vi "VI Server_Set Controls Property from String Formats.vi"(6 "Defer Panel Updates (T)":bool=TRUE, 7 "Property (Value)":T2="Value", 8 "error in (no error)":errorcluster, 9 "New Values":string[](array[string]), 10 "Labels":string[](array[string]), 11 "VI Server Cluster":T1={"Labels"=["Label", "Size", "Font", "Heght", "Width", "Ledding Denominator", "Ledding Nominator", "Label Number", "Microstep Resolution", "X", "Y", "Z", "Italic?", "Underlined?"], "Refs"=[], "VI Ref"=refnum}) -> (0 "error out":errorcluster, 2 "Labels.Text":string[](array[string]), 3 "VI Server Cluster.DUP":T1={"Labels"=["Label", "Size", "Font", "Heght", "Width", "Ledding Denominator", "Ledding Nominator", "Label Number", "Microstep Resolution", "X", "Y", "Z", "Italic?", "Underlined?"], "Refs"=[], "VI Ref"=refnum})   [LabVIEW 2020, in "VI Server Toolkit LV2013.lvlib"]
doc: "Set multiple controls <B>Property</B> from string equivalents.\nList of properties include (if applicable):\n- Value;\n- Format;\n-Format String;\n- Increment;\n-Minimum;\n-Maximum;\n-Precision;\n-Boolean Text;\n-Caption."
uses:
  VI Server Toolkit LV2013.lvlib
  VI Server_TypeDefs/VI Server_RefsCluster.ctl
  VI Server Libraries/VI Server Controls.llb/VI Server_Properties.ctl
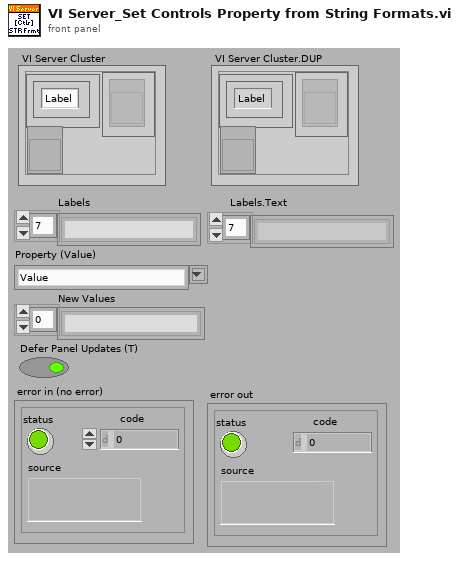
[diagram p1: front panel]
types:
  T1 = typedef "VI Server_RefsCluster.ctl" = cluster{"Labels":string[], "Refs":refnum<vi>[], "VI Ref":refnum<vi>}
  T2 = typedef "VI Server Toolkit LV2013.lvlib/VI Server_Properties.ctl" = string
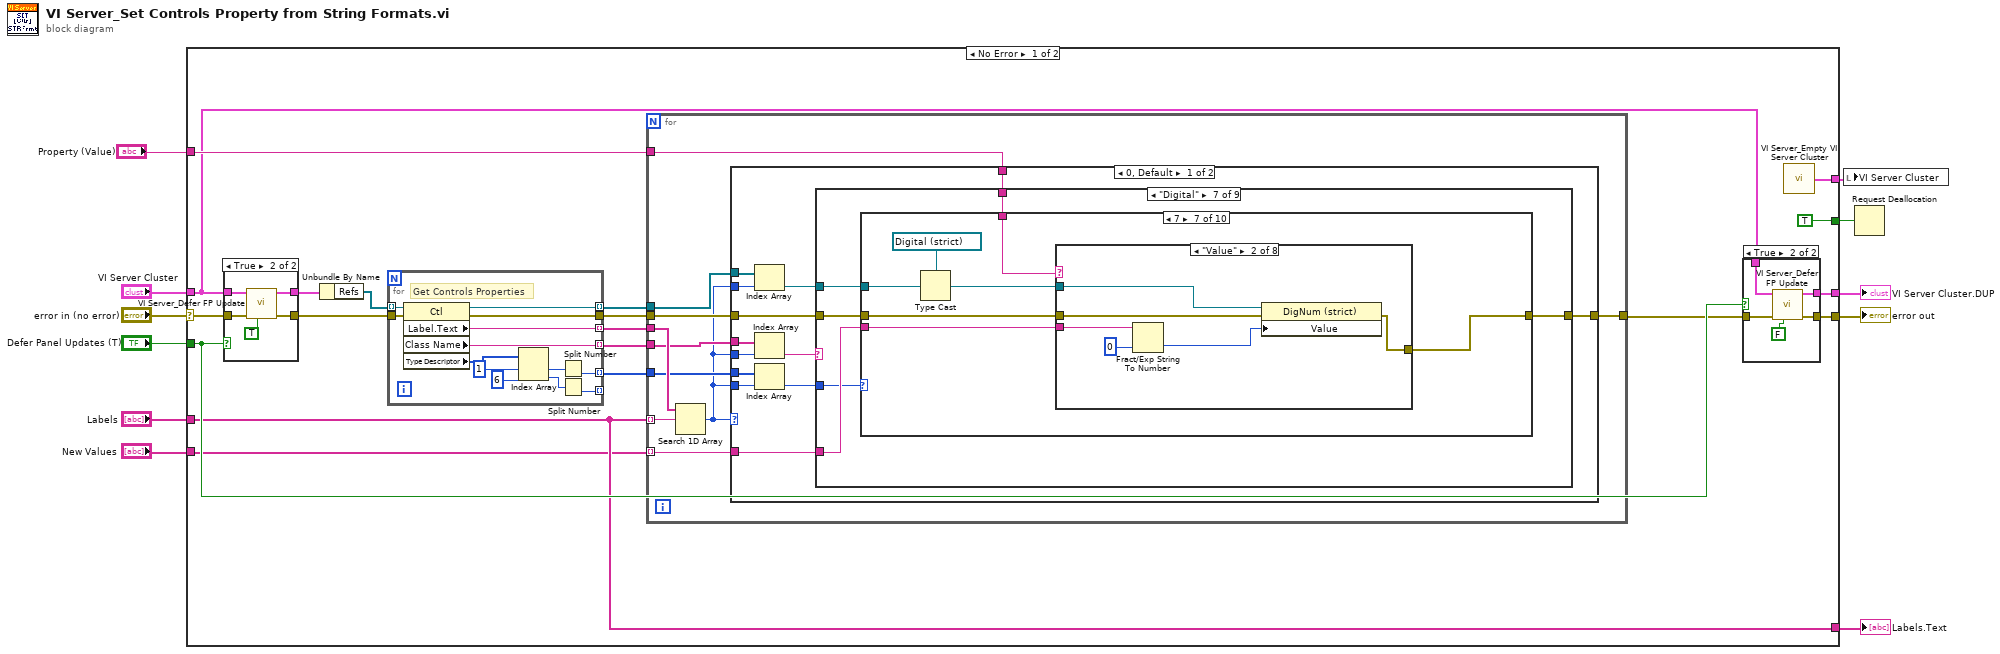
[diagram p0: block diagram]
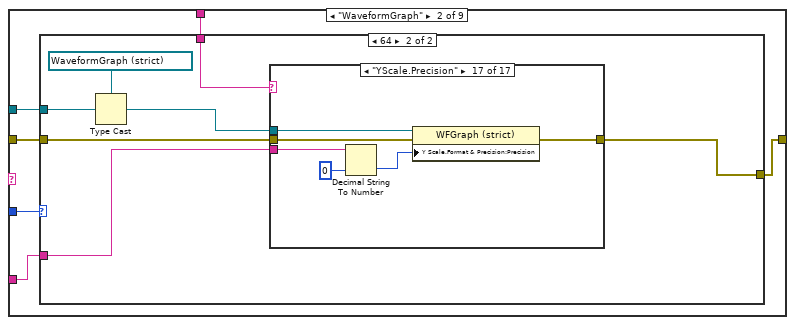
[diagram p3: hidden frame]
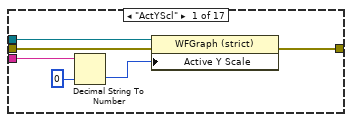
[diagram p5: hidden frame]
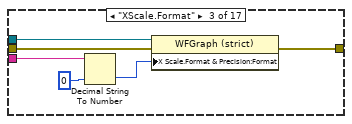
[diagram p7: hidden frame]
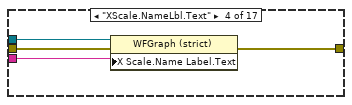
[diagram p8: hidden frame]
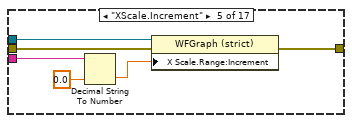
[diagram p9: hidden frame]
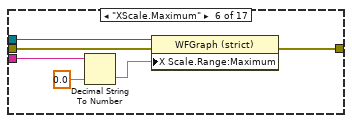
[diagram p10: hidden frame]
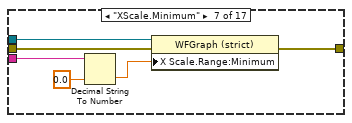
[diagram p11: hidden frame]
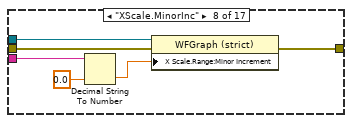
[diagram p12: hidden frame]
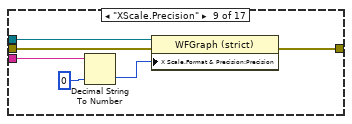
[diagram p13: hidden frame]
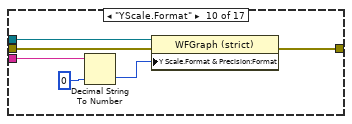
[diagram p14: hidden frame]
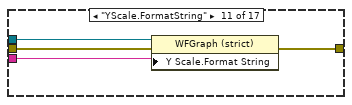
[diagram p15: hidden frame]
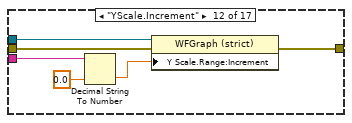
[diagram p16: hidden frame]
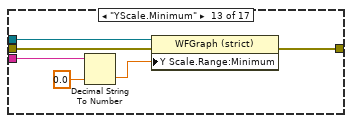
[diagram p17: hidden frame]
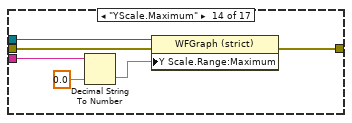
[diagram p18: hidden frame]
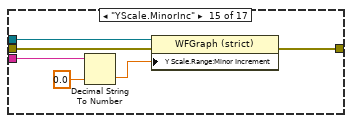
[diagram p19: hidden frame]
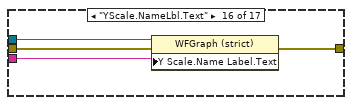
[diagram p20: hidden frame]
diagram:
  n1 = case shown="No Error" "error in (no error)" {
    selector: "error in (no error)" -> [w29 w1413]
    tunnel: "Labels" -> [w15 _]
    tunnel: "New Values" -> [w14 _]
    tunnel: [w26 w1413] -> w9
    tunnel: "VI Server Cluster" -> [w13 _]
    tunnel: "Property (Value)" -> [w19 _]
    tunnel: [w15 _] -> w5
    tunnel: [w25 _] -> w4
    tunnel: "Defer Panel Updates (T)" -> [w24 _]
    tunnel: [TRUE _] -> w2
    tunnel: [w12 _] -> w1
    frame No Error {
      n2 = case shown="True" w24 {
        tunnel: w29 -> [w1394 w1399]
        tunnel: [w1394 w1398] -> w28
        tunnel: w13 -> [w1393 w1397]
        tunnel: [w1393 w1396] -> w27
        frame False {
        }
        frame True {
          n3 = call "VI Server_Defer FP Update.vi"("Defer Panel Updates? (F)"=TRUE ("Defer Panel Updates (F)"), "error in"=w1399, "VI Server Cluster"=w1397) -> ("error out"=w1398:errorcluster, "VI Server Cluster.DUP"=w1396:T1)  [unwired: 7 out]
        }
      }
      n4 = Unbundle By Name(w27) -> ("Refs"=w30:refnum<vi>[])
      n5 = for {
        tunnel: w30 -> [w1412] mode=indexing
        tunnel: w28 -> [w1411]
        tunnel: [w1410] -> w20 mode=indexing
        tunnel: [w1409] -> w17 mode=indexing
        tunnel: [w1408] -> w21 mode=indexing
        tunnel: [w1407] -> w22
        tunnel: [w1403] -> w16 mode=indexing
        tunnel: [w1400] -> _ mode=indexing
        # "Get Controls Properties"
        n6 = property class="Ctl"(reference=w1412, error in=w1411) -> (reference out=w1408:refnum<vi>, error out=w1407:errorcluster, "Label.Text"=w1410:string, "Class Name"=w1409:string, "Type Descriptor"=w1406:i16[])
        n7 = Index Array(array=w1406, index #1=1 ("index"), index #2=6 ("index")) -> (element #1=w1404:i16, element #2=w1401:i16)
        n8 = Split Number(x=w1404) -> (lo(x)=w1403:u8)  [unwired: 1 out]
        n9 = Split Number(x=w1401) -> (lo(x)=w1400:u8)  [unwired: 1 out]
      }
      n10 = for {
        tunnel: w15 -> [w38] mode=indexing
        tunnel: w20 -> [w40]
        tunnel: w21 -> [w36]
        tunnel: w17 -> [w39]
        tunnel: w14 -> [w37] mode=indexing
        tunnel: w22 -> [w35]
        tunnel: [w34] -> w18
        tunnel: w16 -> [w33]
        tunnel: w19 -> [w31]
        n11 = Search 1D Array(1D array=w40, element=w38) -> (index of element=w32:i32)  [unwired: 1 out]
        n12 = case shown="0, Default" w32 {
          tunnel: w36 -> [w53 _]
          tunnel: w32 -> [w52 _]
          tunnel: w39 -> [w51 _]
          tunnel: w32 -> [w50 _]
          tunnel: w37 -> [w47 _]
          tunnel: w35 -> [w46 w1385]
          tunnel: [w45 w1385] -> w34
          tunnel: w33 -> [w44 _]
          tunnel: w32 -> [w43 _]
          tunnel: w31 -> [w41 _]
          frame 0, Default {
            n13 = Index Array(array=w53, index=w52) -> (element=w48:refnum<vi>)
            n14 = Index Array(array=w51, index=w50) -> (element=w49:string)
            n15 = Index Array(array=w44, index=w43) -> (element=w42:u8)
            n16 = case shown="\"Digital\"" w49 {
              tunnel: w48 -> [_ w58 w162 w170 w182 w191 w195 w661 w1371]
              tunnel: w47 -> [_ w56 w167 w178 w185 w189 w194 w660 w1369]
              tunnel: w46 -> [w54 w59 w165 w173 w183 w188 w197 w663 w1373]
              tunnel: [w54 w55 w163 w171 w184 w187 w196 w662 w1372] -> w45
              tunnel: w42 -> [_ w60 _ _ _ _ w193 w659 _]
              tunnel: w41 -> [_ w57 _ _ _ _ w192 w658 w1367]
              frame "", Default {
              }
              frame "WaveformGraph" {
                n17 = case shown="64" w60 {
                  tunnel: w59 -> [w61 w65]
                  tunnel: w58 -> [_ w68]
                  tunnel: w57 -> [_ w64]
                  tunnel: w56 -> [_ w63]
                  tunnel: [w61 w62] -> w55
                  frame 0, Default {
                  }
                  frame 64 {
                    n18 = Type Cast(type=refnum<vi> refnum ("XY Graph"), x=w68) -> (*(type *) &x=w66:refnum<vi>)
                    n19 = case shown="\"YScale.Precision\"" w64 {
                      tunnel: w66 -> [w74 _ w81 w85 w91 w97 w103 w109 w115 w121 w125 w131 w137 w143 w149 w153 w159]
                      tunnel: w65 -> [w73 w75 w80 w84 w90 w96 w102 w108 w114 w120 w124 w130 w136 w142 w148 w152 w158]
                      tunnel: w63 -> [w72 _ w78 w82 w88 w94 w100 w106 w112 w118 w122 w128 w134 w140 w146 w150 w156]
                      tunnel: [w71 w75 w79 w83 w89 w95 w101 w107 w113 w119 w123 w129 w135 w141 w147 w151 w157] -> w62
                      frame "ActYScl" {
                        n20 = Decimal String To Number(string=w72, default (0L)=0 ("Active Y Scale")) -> (number=w69:i32)  [unwired: 2 out]
                        n21 = property class="WFGraph (strict)"(reference=w74, error in=w73, "Active Y Scale"=w69) -> (error out=w71:errorcluster)  [unwired: 1 out]
                      }
                      frame "False", Default {
                      }
                      frame "XScale.Format" {
                        n22 = Decimal String To Number(string=w78, default (0L)=u8 0 ("Y Scale.Format & Precision:Format")) -> (number=w77:u8)  [unwired: 2 out]
                        n23 = property class="WFGraph (strict)"(reference=w81, error in=w80, "X Scale.Format & Precision:Format"=w77) -> (error out=w79:errorcluster)  [unwired: 1 out]
                      }
                      frame "XScale.NameLbl.Text" {
                        n24 = property class="WFGraph (strict)"(reference=w85, error in=w84, "X Scale.Name Label.Text"=w82) -> (error out=w83:errorcluster)  [unwired: 1 out]
                      }
                      frame "XScale.Increment" {
                        n25 = Decimal String To Number(string=w88, default (0L)=0.0 ("X Scale.Range:Minimum")) -> (number=w86:dbl)  [unwired: 2 out]
                        n26 = property class="WFGraph (strict)"(reference=w91, error in=w90, "X Scale.Range:Increment"=w86) -> (error out=w89:errorcluster)  [unwired: 1 out]
                      }
                      frame "XScale.Maximum" {
                        n27 = Decimal String To Number(string=w94, default (0L)=0.0 ("X Scale.Range:Minimum")) -> (number=w92:dbl)  [unwired: 2 out]
                        n28 = property class="WFGraph (strict)"(reference=w97, error in=w96, "X Scale.Range:Maximum"=w92) -> (error out=w95:errorcluster)  [unwired: 1 out]
                      }
                      frame "XScale.Minimum" {
                        n29 = Decimal String To Number(string=w100, default (0L)=0.0 ("X Scale.Range:Minimum")) -> (number=w98:dbl)  [unwired: 2 out]
                        n30 = property class="WFGraph (strict)"(reference=w103, error in=w102, "X Scale.Range:Minimum"=w98) -> (error out=w101:errorcluster)  [unwired: 1 out]
                      }
                      frame "XScale.MinorInc" {
                        n31 = Decimal String To Number(string=w106, default (0L)=0.0 ("X Scale.Range:Minimum")) -> (number=w104:dbl)  [unwired: 2 out]
                        n32 = property class="WFGraph (strict)"(reference=w109, error in=w108, "X Scale.Range:Minor Increment"=w104) -> (error out=w107:errorcluster)  [unwired: 1 out]
                      }
                      frame "XScale.Precision" {
                        n33 = Decimal String To Number(string=w112, default (0L)=u8 0 ("Y Scale.Format & Precision:Format")) -> (number=w111:u8)  [unwired: 2 out]
                        n34 = property class="WFGraph (strict)"(reference=w115, error in=w114, "X Scale.Format & Precision:Precision"=w111) -> (error out=w113:errorcluster)  [unwired: 1 out]
                      }
                      frame "YScale.Format" {
                        n35 = Decimal String To Number(string=w118, default (0L)=u8 0 ("Y Scale.Format & Precision:Format")) -> (number=w117:u8)  [unwired: 2 out]
                        n36 = property class="WFGraph (strict)"(reference=w121, error in=w120, "Y Scale.Format & Precision:Format"=w117) -> (error out=w119:errorcluster)  [unwired: 1 out]
                      }
                      frame "YScale.FormatString" {
                        n37 = property class="WFGraph (strict)"(reference=w125, error in=w124, "Y Scale.Format String"=w122) -> (error out=w123:errorcluster)  [unwired: 1 out]
                      }
                      frame "YScale.Increment" {
                        n38 = Decimal String To Number(string=w128, default (0L)=0.0 ("X Scale.Range:Minimum")) -> (number=w126:dbl)  [unwired: 2 out]
                        n39 = property class="WFGraph (strict)"(reference=w131, error in=w130, "Y Scale.Range:Increment"=w126) -> (error out=w129:errorcluster)  [unwired: 1 out]
                      }
                      frame "YScale.Minimum" {
                        n40 = Decimal String To Number(string=w134, default (0L)=0.0 ("X Scale.Range:Minimum")) -> (number=w132:dbl)  [unwired: 2 out]
                        n41 = property class="WFGraph (strict)"(reference=w137, error in=w136, "Y Scale.Range:Minimum"=w132) -> (error out=w135:errorcluster)  [unwired: 1 out]
                      }
                      frame "YScale.Maximum" {
                        n42 = Decimal String To Number(string=w140, default (0L)=0.0 ("X Scale.Range:Minimum")) -> (number=w138:dbl)  [unwired: 2 out]
                        n43 = property class="WFGraph (strict)"(reference=w143, error in=w142, "Y Scale.Range:Maximum"=w138) -> (error out=w141:errorcluster)  [unwired: 1 out]
                      }
                      frame "YScale.MinorInc" {
                        n44 = Decimal String To Number(string=w146, default (0L)=0.0 ("X Scale.Range:Minimum")) -> (number=w144:dbl)  [unwired: 2 out]
                        n45 = property class="WFGraph (strict)"(reference=w149, error in=w148, "Y Scale.Range:Minor Increment"=w144) -> (error out=w147:errorcluster)  [unwired: 1 out]
                      }
                      frame "YScale.NameLbl.Text" {
                        n46 = property class="WFGraph (strict)"(reference=w153, error in=w152, "Y Scale.Name Label.Text"=w150) -> (error out=w151:errorcluster)  [unwired: 1 out]
                      }
                      frame "YScale.Precision" {
                        n47 = Decimal String To Number(string=w156, default (0L)=u8 0 ("Y Scale.Format & Precision:Format")) -> (number=w155:u8)  [unwired: 2 out]
                        n48 = property class="WFGraph (strict)"(reference=w159, error in=w158, "Y Scale.Format & Precision:Precision"=w155) -> (error out=w157:errorcluster)  [unwired: 1 out]
                      }
                    }
                  }
                }
              }
              frame "Enum" {
                n49 = Type Cast(type=refnum<vi> refnum ("Enum"), x=w162) -> (*(type *) &x=w168:refnum<vi>)
                n50 = property class="Enum (strict)"(reference=w168, error in=w165) -> (error out=w164:errorcluster, "Strings []"=w166:string[])  [unwired: 1 out]
                n51 = Search 1D Array(1D array=w166, element=w167) -> (index of element=w161:i32)  [unwired: 1 out]
                n52 = To Variant(anything=w161) -> (Variant=w160:variant)
                n53 = property class="Ctl"(reference=w162, error in=w164, "Value"=w160) -> (error out=w163:errorcluster)  [unwired: 1 out]
              }
              frame "Ring" {
                n54 = Type Cast(type=refnum<vi> refnum ("Ring"), x=w170) -> (*(type *) &x=w179:refnum<vi>)
                n55 = property class="Ring (strict)"(reference=w179, error in=w173) -> (error out=w172:errorcluster, "Strings []"=w176:string[])  [unwired: 1 out]
                n56 = Search 1D Array(1D array=w176, element=w178) -> (index of element=w177:i32)  [unwired: 1 out]
                n57 = To Variant(anything=w177) -> (Variant=w175:variant)
                n58 = property class="Ctl"(reference=w170, error in=w172, "Value"=w175) -> (error out=w171:errorcluster)  [unwired: 1 out]
              }
              frame "Path" {
                n59 = String To Path(string=w185) -> (path=w186:path)
                n60 = Type Cast(type=refnum<vi> refnum ("Path"), x=w182) -> (*(type *) &x=w181:refnum<vi>)
                n61 = property class="Path"(reference=w181, error in=w183, "Value"=w186) -> (error out=w184:errorcluster)  [unwired: 1 out]
              }
              frame "String" {
                n62 = To Variant(anything=w189) -> (Variant=w190:variant)
                n63 = property class="Ctl"(reference=w191, error in=w188, "Value"=w190) -> (error out=w187:errorcluster)  [unwired: 1 out]
              }
              frame "Digital" {
                n64 = case shown="7" w193 {
                  tunnel: w197 -> [w198 w205 w254 w298 w350 w397 w450 w498 w548 w608]
                  tunnel: [w198 w204 w250 w300 w353 w399 w448 w496 w550 w607] -> w196
                  tunnel: w195 -> [_ w203 w256 w304 w355 w403 w454 w502 w554 w612]
                  tunnel: w194 -> [_ w201 w253 w299 w349 w398 w449 w497 w549 w606]
                  tunnel: w192 -> [_ w199 w252 w302 w352 w401 w452 w499 w552 w610]
                  frame 0, Default {
                  }
                  frame 1 {
                    n65 = Type Cast(type=refnum<vi> refnum ("I8"), x=w203) -> (*(type *) &x=w202:refnum<vi>)
                    n66 = case shown="\"Value\"" w199 {
                      tunnel: w205 -> [w206 w212 w218 w225 w232 w237 w243 w249]
                      tunnel: [w206 w211 w217 w224 w231 w236 w242 w248] -> w204
                      tunnel: w202 -> [_ w210 w216 w223 w230 w235 w241 w247]
                      tunnel: w201 -> [_ w208 w215 w222 w229 w234 w240 w246]
                      frame "False", Default {
                      }
                      frame "Value" {
                        n67 = Fract/Exp String To Number(string=w208, default (0 dbl)=i8 0) -> (number=w207:i8)  [unwired: 3 out]
                        n68 = property class="DigNum (strict)"(reference=w210, error in=w212, "Value"=w207) -> (error out=w211:errorcluster)  [unwired: 1 out]
                      }
                      frame "Minimum" {
                        n69 = Fract/Exp String To Number(string=w215, default (0 dbl)=0.0 ("Data Range:Minimum")) -> (number=w213:dbl)  [unwired: 3 out]
                        n70 = property class="DigNum (strict)"(reference=w216, error in=w218, "Data Range:Minimum"=w213) -> (reference out=w219:refnum<vi>, error out=w217:errorcluster)
                        n71 = Close Reference(reference=w219) -> ()  [unwired: 1 in, 1 out]
                      }
                      frame "Maximum" {
                        n72 = Fract/Exp String To Number(string=w222, default (0 dbl)=0.0 ("Data Range:Minimum")) -> (number=w220:dbl)  [unwired: 3 out]
                        n73 = property class="DigNum (strict)"(reference=w223, error in=w225, "Data Range:Maximum"=w220) -> (reference out=w226:refnum<vi>, error out=w224:errorcluster)
                        n74 = Close Reference(reference=w226) -> ()  [unwired: 1 in, 1 out]
                      }
                      frame "Increment" {
                        n75 = Fract/Exp String To Number(string=w229, default (0 dbl)=0.0 ("Data Range:Minimum")) -> (number=w227:dbl)  [unwired: 3 out]
                        n76 = property class="DigNum (strict)"(reference=w230, error in=w232, "Data Range:Increment"=w227) -> (reference out=w233:refnum<vi>, error out=w231:errorcluster)
                        n77 = Close Reference(reference=w233) -> ()  [unwired: 1 in, 1 out]
                      }
                      frame "Format String" {
                        n78 = property class="DigNum (strict)"(reference=w235, error in=w237, "Format String"=w234) -> (error out=w236:errorcluster)  [unwired: 1 out]
                      }
                      frame "Format" {
                        n79 = Decimal String To Number(string=w240, default (0L)=u8 0 ("Format & Precision:Format")) -> (number=w238:u8)  [unwired: 2 out]
                        n80 = property class="DigNum (strict)"(reference=w241, error in=w243, "Format & Precision:Format"=w238) -> (error out=w242:errorcluster)  [unwired: 1 out]
                      }
                      frame "Precision" {
                        n81 = Decimal String To Number(string=w246, default (0L)=u8 0 ("Format & Precision:Format")) -> (number=w244:u8)  [unwired: 2 out]
                        n82 = property class="DigNum (strict)"(reference=w247, error in=w249, "Format & Precision:Precision"=w244) -> (error out=w248:errorcluster)  [unwired: 1 out]
                      }
                    }
                  }
                  frame 2 {
                    n83 = Type Cast(type=refnum<vi> refnum ("I16"), x=w256) -> (*(type *) &x=w251:refnum<vi>)
                    n84 = case shown="\"Value\"" w252 {
                      tunnel: w254 -> [w257 w263 w269 w275 w281 w285 w291 w297]
                      tunnel: [w257 w262 w268 w274 w280 w284 w290 w296] -> w250
                      tunnel: w251 -> [_ w261 w267 w273 w279 w283 w289 w295]
                      tunnel: w253 -> [_ w260 w266 w272 w278 w282 w288 w294]
                      frame "False", Default {
                      }
                      frame "Value" {
                        n85 = Fract/Exp String To Number(string=w260, default (0 dbl)=i16 0) -> (number=w259:i16)  [unwired: 3 out]
                        n86 = property class="DigNum (strict)"(reference=w261, error in=w263, "Value"=w259) -> (error out=w262:errorcluster)  [unwired: 1 out]
                      }
                      frame "Minimum" {
                        n87 = Fract/Exp String To Number(string=w266, default (0 dbl)=0.0 ("Data Range:Minimum")) -> (number=w264:dbl)  [unwired: 3 out]
                        n88 = property class="DigNum (strict)"(reference=w267, error in=w269, "Data Range:Minimum"=w264) -> (error out=w268:errorcluster)  [unwired: 1 out]
                      }
                      frame "Maximum" {
                        n89 = Fract/Exp String To Number(string=w272, default (0 dbl)=0.0 ("Data Range:Minimum")) -> (number=w270:dbl)  [unwired: 3 out]
                        n90 = property class="DigNum (strict)"(reference=w273, error in=w275, "Data Range:Maximum"=w270) -> (error out=w274:errorcluster)  [unwired: 1 out]
                      }
                      frame "Increment" {
                        n91 = Fract/Exp String To Number(string=w278, default (0 dbl)=0.0 ("Data Range:Minimum")) -> (number=w276:dbl)  [unwired: 3 out]
                        n92 = property class="DigNum (strict)"(reference=w279, error in=w281, "Data Range:Increment"=w276) -> (error out=w280:errorcluster)  [unwired: 1 out]
                      }
                      frame "Format String" {
                        n93 = property class="DigNum (strict)"(reference=w283, error in=w285, "Format String"=w282) -> (error out=w284:errorcluster)  [unwired: 1 out]
                      }
                      frame "Format" {
                        n94 = Decimal String To Number(string=w288, default (0L)=u8 0 ("Format & Precision:Format")) -> (number=w286:u8)  [unwired: 2 out]
                        n95 = property class="DigNum (strict)"(reference=w289, error in=w291, "Format & Precision:Format"=w286) -> (error out=w290:errorcluster)  [unwired: 1 out]
                      }
                      frame "Precision" {
                        n96 = Decimal String To Number(string=w294, default (0L)=u8 0 ("Format & Precision:Format")) -> (number=w292:u8)  [unwired: 2 out]
                        n97 = property class="DigNum (strict)"(reference=w295, error in=w297, "Format & Precision:Precision"=w292) -> (error out=w296:errorcluster)  [unwired: 1 out]
                      }
                    }
                  }
                  frame 3 {
                    n98 = Type Cast(type=refnum<vi> refnum ("I32"), x=w304) -> (*(type *) &x=w301:refnum<vi>)
                    n99 = case shown="\"Value\"" w302 {
                      tunnel: w298 -> [w305 w311 w317 w324 w331 w336 w342 w348]
                      tunnel: [w305 w310 w316 w323 w330 w335 w341 w347] -> w300
                      tunnel: w301 -> [_ w309 w315 w322 w329 w334 w340 w346]
                      tunnel: w299 -> [_ w308 w314 w321 w328 w333 w339 w345]
                      frame "False", Default {
                      }
                      frame "Value" {
                        n100 = Fract/Exp String To Number(string=w308, default (0 dbl)=0) -> (number=w307:i32)  [unwired: 3 out]
                        n101 = property class="DigNum (strict)"(reference=w309, error in=w311, "Value"=w307) -> (error out=w310:errorcluster)  [unwired: 1 out]
                      }
                      frame "Minimum" {
                        n102 = Fract/Exp String To Number(string=w314, default (0 dbl)=0.0 ("Data Range:Minimum")) -> (number=w312:dbl)  [unwired: 3 out]
                        n103 = property class="DigNum (strict)"(reference=w315, error in=w317, "Data Range:Minimum"=w312) -> (reference out=w318:refnum<vi>, error out=w316:errorcluster)
                        n104 = Close Reference(reference=w318) -> ()  [unwired: 1 in, 1 out]
                      }
                      frame "Maximum" {
                        n105 = Fract/Exp String To Number(string=w321, default (0 dbl)=0.0 ("Data Range:Minimum")) -> (number=w319:dbl)  [unwired: 3 out]
                        n106 = property class="DigNum (strict)"(reference=w322, error in=w324, "Data Range:Maximum"=w319) -> (reference out=w325:refnum<vi>, error out=w323:errorcluster)
                        n107 = Close Reference(reference=w325) -> ()  [unwired: 1 in, 1 out]
                      }
                      frame "Increment" {
                        n108 = Fract/Exp String To Number(string=w328, default (0 dbl)=0.0 ("Data Range:Minimum")) -> (number=w326:dbl)  [unwired: 3 out]
                        n109 = property class="DigNum (strict)"(reference=w329, error in=w331, "Data Range:Increment"=w326) -> (reference out=w332:refnum<vi>, error out=w330:errorcluster)
                        n110 = Close Reference(reference=w332) -> ()  [unwired: 1 in, 1 out]
                      }
                      frame "Format String" {
                        n111 = property class="DigNum (strict)"(reference=w334, error in=w336, "Format String"=w333) -> (error out=w335:errorcluster)  [unwired: 1 out]
                      }
                      frame "Format" {
                        n112 = Decimal String To Number(string=w339, default (0L)=u8 0 ("Format & Precision:Format")) -> (number=w337:u8)  [unwired: 2 out]
                        n113 = property class="DigNum (strict)"(reference=w340, error in=w342, "Format & Precision:Format"=w337) -> (error out=w341:errorcluster)  [unwired: 1 out]
                      }
                      frame "Precision" {
                        n114 = Decimal String To Number(string=w345, default (0L)=u8 0 ("Format & Precision:Format")) -> (number=w343:u8)  [unwired: 2 out]
                        n115 = property class="DigNum (strict)"(reference=w346, error in=w348, "Format & Precision:Precision"=w343) -> (error out=w347:errorcluster)  [unwired: 1 out]
                      }
                    }
                  }
                  frame 5 {
                    n116 = Type Cast(type=refnum<vi> refnum ("U8"), x=w355) -> (*(type *) &x=w351:refnum<vi>)
                    n117 = case shown="\"Value\"" w352 {
                      tunnel: w350 -> [w356 w362 w368 w374 w380 w384 w390 w396]
                      tunnel: [w356 w361 w367 w373 w379 w383 w389 w395] -> w353
                      tunnel: w351 -> [_ w360 w366 w372 w378 w382 w388 w394]
                      tunnel: w349 -> [_ w359 w365 w371 w377 w381 w387 w393]
                      frame "False", Default {
                      }
                      frame "Value" {
                        n118 = Fract/Exp String To Number(string=w359, default (0 dbl)=u8 0) -> (number=w358:u8)  [unwired: 3 out]
                        n119 = property class="DigNum (strict)"(reference=w360, error in=w362, "Value"=w358) -> (error out=w361:errorcluster)  [unwired: 1 out]
                      }
                      frame "Minimum" {
                        n120 = Fract/Exp String To Number(string=w365, default (0 dbl)=0.0 ("Data Range:Minimum")) -> (number=w363:dbl)  [unwired: 3 out]
                        n121 = property class="DigNum (strict)"(reference=w366, error in=w368, "Data Range:Minimum"=w363) -> (error out=w367:errorcluster)  [unwired: 1 out]
                      }
                      frame "Maximum" {
                        n122 = Fract/Exp String To Number(string=w371, default (0 dbl)=0.0 ("Data Range:Minimum")) -> (number=w369:dbl)  [unwired: 3 out]
                        n123 = property class="DigNum (strict)"(reference=w372, error in=w374, "Data Range:Maximum"=w369) -> (error out=w373:errorcluster)  [unwired: 1 out]
                      }
                      frame "Increment" {
                        n124 = Fract/Exp String To Number(string=w377, default (0 dbl)=0.0 ("Data Range:Minimum")) -> (number=w375:dbl)  [unwired: 3 out]
                        n125 = property class="DigNum (strict)"(reference=w378, error in=w380, "Data Range:Increment"=w375) -> (error out=w379:errorcluster)  [unwired: 1 out]
                      }
                      frame "Format String" {
                        n126 = property class="DigNum (strict)"(reference=w382, error in=w384, "Format String"=w381) -> (error out=w383:errorcluster)  [unwired: 1 out]
                      }
                      frame "Format" {
                        n127 = Decimal String To Number(string=w387, default (0L)=u8 0 ("Format & Precision:Format")) -> (number=w385:u8)  [unwired: 2 out]
                        n128 = property class="DigNum (strict)"(reference=w388, error in=w390, "Format & Precision:Format"=w385) -> (error out=w389:errorcluster)  [unwired: 1 out]
                      }
                      frame "Precision" {
                        n129 = Decimal String To Number(string=w393, default (0L)=u8 0 ("Format & Precision:Format")) -> (number=w391:u8)  [unwired: 2 out]
                        n130 = property class="DigNum (strict)"(reference=w394, error in=w396, "Format & Precision:Precision"=w391) -> (error out=w395:errorcluster)  [unwired: 1 out]
                      }
                    }
                  }
                  frame 6 {
                    n131 = Type Cast(type=refnum<vi> refnum ("U16"), x=w403) -> (*(type *) &x=w400:refnum<vi>)
                    n132 = case shown="\"Value\"" w401 {
                      tunnel: w397 -> [w404 w410 w416 w423 w430 w435 w441 w447]
                      tunnel: [w404 w409 w415 w422 w429 w434 w440 w446] -> w399
                      tunnel: w400 -> [_ w408 w414 w421 w428 w433 w439 w445]
                      tunnel: w398 -> [_ w407 w413 w420 w427 w432 w438 w444]
                      frame "False", Default {
                      }
                      frame "Value" {
                        n133 = Fract/Exp String To Number(string=w407, default (0 dbl)=u16 0) -> (number=w406:u16)  [unwired: 3 out]
                        n134 = property class="DigNum (strict)"(reference=w408, error in=w410, "Value"=w406) -> (error out=w409:errorcluster)  [unwired: 1 out]
                      }
                      frame "Minimum" {
                        n135 = Fract/Exp String To Number(string=w413, default (0 dbl)=0.0 ("Data Range:Minimum")) -> (number=w411:dbl)  [unwired: 3 out]
                        n136 = property class="DigNum (strict)"(reference=w414, error in=w416, "Data Range:Minimum"=w411) -> (reference out=w417:refnum<vi>, error out=w415:errorcluster)
                        n137 = Close Reference(reference=w417) -> ()  [unwired: 1 in, 1 out]
                      }
                      frame "Maximum" {
                        n138 = Fract/Exp String To Number(string=w420, default (0 dbl)=0.0 ("Data Range:Minimum")) -> (number=w418:dbl)  [unwired: 3 out]
                        n139 = property class="DigNum (strict)"(reference=w421, error in=w423, "Data Range:Maximum"=w418) -> (reference out=w424:refnum<vi>, error out=w422:errorcluster)
                        n140 = Close Reference(reference=w424) -> ()  [unwired: 1 in, 1 out]
                      }
                      frame "Increment" {
                        n141 = Fract/Exp String To Number(string=w427, default (0 dbl)=0.0 ("Data Range:Minimum")) -> (number=w425:dbl)  [unwired: 3 out]
                        n142 = property class="DigNum (strict)"(reference=w428, error in=w430, "Data Range:Increment"=w425) -> (reference out=w431:refnum<vi>, error out=w429:errorcluster)
                        n143 = Close Reference(reference=w431) -> ()  [unwired: 1 in, 1 out]
                      }
                      frame "Format String" {
                        n144 = property class="DigNum (strict)"(reference=w433, error in=w435, "Format String"=w432) -> (error out=w434:errorcluster)  [unwired: 1 out]
                      }
                      frame "Format" {
                        n145 = Decimal String To Number(string=w438, default (0L)=u8 0 ("Format & Precision:Format")) -> (number=w436:u8)  [unwired: 2 out]
                        n146 = property class="DigNum (strict)"(reference=w439, error in=w441, "Format & Precision:Format"=w436) -> (error out=w440:errorcluster)  [unwired: 1 out]
                      }
                      frame "Precision" {
                        n147 = Decimal String To Number(string=w444, default (0L)=u8 0 ("Format & Precision:Format")) -> (number=w442:u8)  [unwired: 2 out]
                        n148 = property class="DigNum (strict)"(reference=w445, error in=w447, "Format & Precision:Precision"=w442) -> (error out=w446:errorcluster)  [unwired: 1 out]
                      }
                    }
                  }
                  frame 7 {
                    n149 = Type Cast(type=refnum<vi> refnum ("U32"), x=w454) -> (*(type *) &x=w451:refnum<vi>)
                    n150 = case shown="\"Value\"" w452 {
                      tunnel: w450 -> [w455 w461 w467 w473 w479 w483 w489 w495]
                      tunnel: [w455 w460 w466 w472 w478 w482 w488 w494] -> w448
                      tunnel: w451 -> [_ w459 w465 w471 w477 w481 w487 w493]
                      tunnel: w449 -> [_ w458 w464 w470 w476 w480 w486 w492]
                      frame "False", Default {
                      }
                      frame "Value" {
                        n151 = Fract/Exp String To Number(string=w458, default (0 dbl)=u32 0) -> (number=w457:u32)  [unwired: 3 out]
                        n152 = property class="DigNum (strict)"(reference=w459, error in=w461, "Value"=w457) -> (error out=w460:errorcluster)  [unwired: 1 out]
                      }
                      frame "Minimum" {
                        n153 = Fract/Exp String To Number(string=w464, default (0 dbl)=0.0 ("Data Range:Minimum")) -> (number=w462:dbl)  [unwired: 3 out]
                        n154 = property class="DigNum (strict)"(reference=w465, error in=w467, "Data Range:Minimum"=w462) -> (error out=w466:errorcluster)  [unwired: 1 out]
                      }
                      frame "Maximum" {
                        n155 = Fract/Exp String To Number(string=w470, default (0 dbl)=0.0 ("Data Range:Minimum")) -> (number=w468:dbl)  [unwired: 3 out]
                        n156 = property class="DigNum (strict)"(reference=w471, error in=w473, "Data Range:Maximum"=w468) -> (error out=w472:errorcluster)  [unwired: 1 out]
                      }
                      frame "Increment" {
                        n157 = Fract/Exp String To Number(string=w476, default (0 dbl)=0.0 ("Data Range:Minimum")) -> (number=w474:dbl)  [unwired: 3 out]
                        n158 = property class="DigNum (strict)"(reference=w477, error in=w479, "Data Range:Increment"=w474) -> (error out=w478:errorcluster)  [unwired: 1 out]
                      }
                      frame "Format String" {
                        n159 = property class="DigNum (strict)"(reference=w481, error in=w483, "Format String"=w480) -> (error out=w482:errorcluster)  [unwired: 1 out]
                      }
                      frame "Format" {
                        n160 = Decimal String To Number(string=w486, default (0L)=u8 0 ("Format & Precision:Format")) -> (number=w484:u8)  [unwired: 2 out]
                        n161 = property class="DigNum (strict)"(reference=w487, error in=w489, "Format & Precision:Format"=w484) -> (error out=w488:errorcluster)  [unwired: 1 out]
                      }
                      frame "Precision" {
                        n162 = Decimal String To Number(string=w492, default (0L)=u8 0 ("Format & Precision:Format")) -> (number=w490:u8)  [unwired: 2 out]
                        n163 = property class="DigNum (strict)"(reference=w493, error in=w495, "Format & Precision:Precision"=w490) -> (error out=w494:errorcluster)  [unwired: 1 out]
                      }
                    }
                  }
                  frame 9 {
                    n164 = Type Cast(type=refnum<vi> refnum ("SGL"), x=w502) -> (*(type *) &x=w500:refnum<vi>)
                    n165 = case shown="\"Value\"" w499 {
                      tunnel: w498 -> [w503 w513 w519 w525 w531 w535 w541 w547]
                      tunnel: [w503 w512 w518 w524 w530 w534 w540 w546] -> w496
                      tunnel: w500 -> [_ w511 w517 w523 w529 w533 w539 w545]
                      tunnel: w497 -> [_ w506 w516 w522 w528 w532 w538 w544]
                      frame "False", Default {
                      }
                      frame "Value" {
                        n166 = Empty String/Path?(string/path=w506) -> (empty?=w509:bool)
                        n167 = Not(x=w509) -> (.not. x?=w508:bool)
                        n168 = Fract/Exp String To Number(string=w506, default (0 dbl)=sgl 0.0) -> (number=w505:sgl)  [unwired: 3 out]
                        n169 = Select(t=w505, s=w508, f=sgl nan) -> (s? t:f=w504:sgl)
                        n170 = property class="DigNum (strict)"(reference=w511, error in=w513, "Value"=w504) -> (error out=w512:errorcluster)  [unwired: 1 out]
                      }
                      frame "Minimum" {
                        n171 = Fract/Exp String To Number(string=w516, default (0 dbl)=0.0 ("Data Range:Minimum")) -> (number=w514:dbl)  [unwired: 3 out]
                        n172 = property class="DigNum (strict)"(reference=w517, error in=w519, "Data Range:Minimum"=w514) -> (error out=w518:errorcluster)  [unwired: 1 out]
                      }
                      frame "Maximum" {
                        n173 = Fract/Exp String To Number(string=w522, default (0 dbl)=0.0 ("Data Range:Minimum")) -> (number=w520:dbl)  [unwired: 3 out]
                        n174 = property class="DigNum (strict)"(reference=w523, error in=w525, "Data Range:Maximum"=w520) -> (error out=w524:errorcluster)  [unwired: 1 out]
                      }
                      frame "Increment" {
                        n175 = Fract/Exp String To Number(string=w528, default (0 dbl)=0.0 ("Data Range:Minimum")) -> (number=w526:dbl)  [unwired: 3 out]
                        n176 = property class="DigNum (strict)"(reference=w529, error in=w531, "Data Range:Increment"=w526) -> (error out=w530:errorcluster)  [unwired: 1 out]
                      }
                      frame "Format String" {
                        n177 = property class="DigNum (strict)"(reference=w533, error in=w535, "Format String"=w532) -> (error out=w534:errorcluster)  [unwired: 1 out]
                      }
                      frame "Format" {
                        n178 = Decimal String To Number(string=w538, default (0L)=u8 0 ("Format & Precision:Format")) -> (number=w536:u8)  [unwired: 2 out]
                        n179 = property class="DigNum (strict)"(reference=w539, error in=w541, "Format & Precision:Format"=w536) -> (error out=w540:errorcluster)  [unwired: 1 out]
                      }
                      frame "Precision" {
                        n180 = Decimal String To Number(string=w544, default (0L)=u8 0 ("Format & Precision:Format")) -> (number=w542:u8)  [unwired: 2 out]
                        n181 = property class="DigNum (strict)"(reference=w545, error in=w547, "Format & Precision:Precision"=w542) -> (error out=w546:errorcluster)  [unwired: 1 out]
                      }
                    }
                  }
                  frame 10 {
                    n182 = Type Cast(type=refnum<vi> refnum ("DBL"), x=w554) -> (*(type *) &x=w551:refnum<vi>)
                    n183 = case shown="\"Value\"" w552 {
                      tunnel: w548 -> [w555 w561 w566 w573 w580 w587 w594 w605]
                      tunnel: [w555 w560 w565 w572 w579 w586 w593 w604] -> w550
                      tunnel: w551 -> [_ w559 w564 w571 w578 w585 w592 w603]
                      tunnel: w549 -> [_ w558 w563 w570 w577 w584 w591 w601]
                      frame "False", Default {
                      }
                      frame "Format" {
                        n184 = Decimal String To Number(string=w558, default (0L)=u8 0 ("Format & Precision:Format")) -> (number=w556:u8)  [unwired: 2 out]
                        n185 = property class="DigNum (strict)"(reference=w559, error in=w561, "Format & Precision:Format"=w556) -> (reference out=w562:refnum<vi>, error out=w560:errorcluster)
                        n186 = Close Reference(reference=w562) -> ()  [unwired: 1 in, 1 out]
                      }
                      frame "Format String" {
                        n187 = property class="DigNum (strict)"(reference=w564, error in=w566, "Format String"=w563) -> (reference out=w567:refnum<vi>, error out=w565:errorcluster)
                        n188 = Close Reference(reference=w567) -> ()  [unwired: 1 in, 1 out]
                      }
                      frame "Increment" {
                        n189 = Fract/Exp String To Number(string=w570, default (0 dbl)=0.0 ("Data Range:Minimum")) -> (number=w568:dbl)  [unwired: 3 out]
                        n190 = property class="DigNum (strict)"(reference=w571, error in=w573, "Data Range:Increment"=w568) -> (reference out=w574:refnum<vi>, error out=w572:errorcluster)
                        n191 = Close Reference(reference=w574) -> ()  [unwired: 1 in, 1 out]
                      }
                      frame "Maximum" {
                        n192 = Fract/Exp String To Number(string=w577, default (0 dbl)=0.0 ("Data Range:Minimum")) -> (number=w575:dbl)  [unwired: 3 out]
                        n193 = property class="DigNum (strict)"(reference=w578, error in=w580, "Data Range:Maximum"=w575) -> (reference out=w581:refnum<vi>, error out=w579:errorcluster)
                        n194 = Close Reference(reference=w581) -> ()  [unwired: 1 in, 1 out]
                      }
                      frame "Minimum" {
                        n195 = Fract/Exp String To Number(string=w584, default (0 dbl)=0.0 ("Data Range:Minimum")) -> (number=w582:dbl)  [unwired: 3 out]
                        n196 = property class="DigNum (strict)"(reference=w585, error in=w587, "Data Range:Minimum"=w582) -> (reference out=w588:refnum<vi>, error out=w586:errorcluster)
                        n197 = Close Reference(reference=w588) -> ()  [unwired: 1 in, 1 out]
                      }
                      frame "Precision" {
                        n198 = Decimal String To Number(string=w591, default (0L)=u8 0 ("Format & Precision:Format")) -> (number=w589:u8)  [unwired: 2 out]
                        n199 = property class="DigNum (strict)"(reference=w592, error in=w594, "Format & Precision:Precision"=w589) -> (reference out=w595:refnum<vi>, error out=w593:errorcluster)
                        n200 = Close Reference(reference=w595) -> ()  [unwired: 1 in, 1 out]
                      }
                      frame "Value" {
                        n201 = Empty String/Path?(string/path=w601) -> (empty?=w600:bool)
                        n202 = Not(x=w600) -> (.not. x?=w599:bool)
                        n203 = Fract/Exp String To Number(string=w601, default (0 dbl)=0.0) -> (number=w598:dbl)  [unwired: 3 out]
                        n204 = Select(t=w598, s=w599, f=nan) -> (s? t:f=w597:dbl)
                        n205 = property class="DigNum (strict)"(reference=w603, error in=w605, "Value"=w597) -> (error out=w604:errorcluster)  [unwired: 1 out]
                      }
                    }
                  }
                  frame 11 {
                    n206 = Type Cast(type=refnum<vi> refnum ("EXT"), x=w612) -> (*(type *) &x=w609:refnum<vi>)
                    n207 = case shown="\"Value\"" w610 {
                      tunnel: w608 -> [w613 w623 w629 w635 w641 w645 w651 w657]
                      tunnel: [w613 w622 w628 w634 w640 w644 w650 w656] -> w607
                      tunnel: w609 -> [_ w621 w627 w633 w639 w643 w649 w655]
                      tunnel: w606 -> [_ w616 w626 w632 w638 w642 w648 w654]
                      frame "False", Default {
                      }
                      frame "Value" {
                        n208 = Empty String/Path?(string/path=w616) -> (empty?=w619:bool)
                        n209 = Not(x=w619) -> (.not. x?=w618:bool)
                        n210 = Fract/Exp String To Number(string=w616, default (0 dbl)=ext 0.0) -> (number=w615:ext)  [unwired: 3 out]
                        n211 = Select(t=w615, s=w618, f=ext nan) -> (s? t:f=w614:ext)
                        n212 = property class="DigNum (strict)"(reference=w621, error in=w623, "Value"=w614) -> (error out=w622:errorcluster)  [unwired: 1 out]
                      }
                      frame "Minimum" {
                        n213 = Fract/Exp String To Number(string=w626, default (0 dbl)=0.0 ("Data Range:Minimum")) -> (number=w624:dbl)  [unwired: 3 out]
                        n214 = property class="DigNum (strict)"(reference=w627, error in=w629, "Data Range:Minimum"=w624) -> (error out=w628:errorcluster)  [unwired: 1 out]
                      }
                      frame "Maximum" {
                        n215 = Fract/Exp String To Number(string=w632, default (0 dbl)=0.0 ("Data Range:Minimum")) -> (number=w630:dbl)  [unwired: 3 out]
                        n216 = property class="DigNum (strict)"(reference=w633, error in=w635, "Data Range:Maximum"=w630) -> (error out=w634:errorcluster)  [unwired: 1 out]
                      }
                      frame "Increment" {
                        n217 = Fract/Exp String To Number(string=w638, default (0 dbl)=0.0 ("Data Range:Minimum")) -> (number=w636:dbl)  [unwired: 3 out]
                        n218 = property class="DigNum (strict)"(reference=w639, error in=w641, "Data Range:Increment"=w636) -> (error out=w640:errorcluster)  [unwired: 1 out]
                      }
                      frame "Format String" {
                        n219 = property class="DigNum (strict)"(reference=w643, error in=w645, "Format String"=w642) -> (error out=w644:errorcluster)  [unwired: 1 out]
                      }
                      frame "Format" {
                        n220 = Decimal String To Number(string=w648, default (0L)=u8 0 ("Format & Precision:Format")) -> (number=w646:u8)  [unwired: 2 out]
                        n221 = property class="DigNum (strict)"(reference=w649, error in=w651, "Format & Precision:Format"=w646) -> (error out=w650:errorcluster)  [unwired: 1 out]
                      }
                      frame "Precision" {
                        n222 = Decimal String To Number(string=w654, default (0L)=u8 0 ("Format & Precision:Format")) -> (number=w652:u8)  [unwired: 2 out]
                        n223 = property class="DigNum (strict)"(reference=w655, error in=w657, "Format & Precision:Precision"=w652) -> (error out=w656:errorcluster)  [unwired: 1 out]
                      }
                    }
                  }
                }
              }
              frame "Slide" {
                n224 = case shown="2" w659 {
                  tunnel: w663 -> [w664 w667 w745 w823 w901 w981 w1056 w1135 w1212 w1291]
                  tunnel: [w664 w665 w743 w821 w902 w982 w1059 w1133 w1213 w1289] -> w662
                  tunnel: w661 -> [_ w671 w749 w827 w905 w983 w1061 w1139 w1217 w1295]
                  tunnel: w660 -> [_ w666 w744 w822 w900 w978 w1055 w1134 w1211 w1290]
                  tunnel: w658 -> [_ w669 w747 w825 w904 w979 w1058 w1137 w1215 w1293]
                  frame 0, Default {
                  }
                  frame 9 {
                    n225 = Type Cast(type=refnum<vi> refnum ("Slide"), x=w671) -> (*(type *) &x=w668:refnum<vi>)
                    n226 = case shown="\"Value\"" w669 {
                      tunnel: w667 -> [w672 w678 w684 w690 w696 w702 w708 w714 w720 w726 w730 w736 w742]
                      tunnel: [w672 w677 w683 w689 w695 w701 w707 w713 w719 w725 w729 w735 w741] -> w665
                      tunnel: w668 -> [_ w676 w682 w688 w694 w700 w706 w712 w718 w724 w728 w734 w740]
                      tunnel: w666 -> [_ w675 w681 w687 w693 w699 w705 w711 w717 w723 w727 w733 w739]
                      frame "False", Default {
                      }
                      frame "Value" {
                        n227 = Fract/Exp String To Number(string=w675, default (0 dbl)=sgl 0.0) -> (number=w674:sgl)  [unwired: 3 out]
                        n228 = property class="Slide (strict)"(reference=w676, error in=w678, "Value"=w674) -> (error out=w677:errorcluster)  [unwired: 1 out]
                      }
                      frame "Minimum" {
                        n229 = Fract/Exp String To Number(string=w681, default (0 dbl)=0.0 ("Data Range:Minimum")) -> (number=w679:dbl)  [unwired: 3 out]
                        n230 = property class="Slide (strict)"(reference=w682, error in=w684, "Data Range:Minimum"=w679) -> (error out=w683:errorcluster)  [unwired: 1 out]
                      }
                      frame "Scale.Minimum" {
                        n231 = Fract/Exp String To Number(string=w687, default (0 dbl)=0.0 ("Data Range:Minimum")) -> (number=w685:dbl)  [unwired: 3 out]
                        n232 = property class="Slide (strict)"(reference=w688, error in=w690, "Scale.Range:Minimum"=w685) -> (error out=w689:errorcluster)  [unwired: 1 out]
                      }
                      frame "Maximum" {
                        n233 = Fract/Exp String To Number(string=w693, default (0 dbl)=0.0 ("Data Range:Minimum")) -> (number=w691:dbl)  [unwired: 3 out]
                        n234 = property class="Slide (strict)"(reference=w694, error in=w696, "Data Range:Maximum"=w691) -> (error out=w695:errorcluster)  [unwired: 1 out]
                      }
                      frame "Scale.Maximum" {
                        n235 = Fract/Exp String To Number(string=w699, default (0 dbl)=0.0 ("Data Range:Minimum")) -> (number=w697:dbl)  [unwired: 3 out]
                        n236 = property class="Slide (strict)"(reference=w700, error in=w702, "Scale.Range:Maximum"=w697) -> (error out=w701:errorcluster)  [unwired: 1 out]
                      }
                      frame "Increment" {
                        n237 = Fract/Exp String To Number(string=w705, default (0 dbl)=0.0 ("Data Range:Minimum")) -> (number=w703:dbl)  [unwired: 3 out]
                        n238 = property class="Slide (strict)"(reference=w706, error in=w708, "Data Range:Increment"=w703) -> (error out=w707:errorcluster)  [unwired: 1 out]
                      }
                      frame "Scale.Increment" {
                        n239 = Fract/Exp String To Number(string=w711, default (0 dbl)=0.0 ("Data Range:Minimum")) -> (number=w709:dbl)  [unwired: 3 out]
                        n240 = property class="Slide (strict)"(reference=w712, error in=w714, "Scale.Range:Increment"=w709) -> (error out=w713:errorcluster)  [unwired: 1 out]
                      }
                      frame "Scale.Start" {
                        n241 = Fract/Exp String To Number(string=w717, default (0 dbl)=0.0 ("Data Range:Minimum")) -> (number=w715:dbl)  [unwired: 3 out]
                        n242 = property class="Slide (strict)"(reference=w718, error in=w720, "Scale.Range:Start"=w715) -> (error out=w719:errorcluster)  [unwired: 1 out]
                      }
                      frame "Scale.MinorInc" {
                        n243 = Fract/Exp String To Number(string=w723, default (0 dbl)=0.0 ("Data Range:Minimum")) -> (number=w721:dbl)  [unwired: 3 out]
                        n244 = property class="Slide (strict)"(reference=w724, error in=w726, "Scale.Range:Minor Increment"=w721) -> (error out=w725:errorcluster)  [unwired: 1 out]
                      }
                      frame "Scale.Format String" {
                        n245 = property class="Slide (strict)"(reference=w728, error in=w730, "Scale.Format String"=w727) -> (error out=w729:errorcluster)  [unwired: 1 out]
                      }
                      frame "Scale.Format" {
                        n246 = Decimal String To Number(string=w733, default (0L)=u8 0 ("Format & Precision:Format")) -> (number=w731:u8)  [unwired: 2 out]
                        n247 = property class="Slide (strict)"(reference=w734, error in=w736, "Scale.Format & Precision:Format"=w731) -> (error out=w735:errorcluster)  [unwired: 1 out]
                      }
                      frame "Scale.Precision" {
                        n248 = Decimal String To Number(string=w739, default (0L)=u8 0 ("Format & Precision:Format")) -> (number=w737:u8)  [unwired: 2 out]
                        n249 = property class="Slide (strict)"(reference=w740, error in=w742, "Scale.Format & Precision:Precision"=w737) -> (error out=w741:errorcluster)  [unwired: 1 out]
                      }
                    }
                  }
                  frame 10 {
                    n250 = Type Cast(type=refnum<vi> refnum ("Slide"), x=w749) -> (*(type *) &x=w746:refnum<vi>)
                    n251 = case shown="\"Value\"" w747 {
                      tunnel: w745 -> [w750 w756 w762 w768 w774 w780 w786 w792 w798 w804 w808 w814 w820]
                      tunnel: [w750 w755 w761 w767 w773 w779 w785 w791 w797 w803 w807 w813 w819] -> w743
                      tunnel: w746 -> [_ w754 w760 w766 w772 w778 w784 w790 w796 w802 w806 w812 w818]
                      tunnel: w744 -> [_ w753 w759 w765 w771 w777 w783 w789 w795 w801 w805 w811 w817]
                      frame "False", Default {
                      }
                      frame "Value" {
                        n252 = Fract/Exp String To Number(string=w753, default (0 dbl)=0.0) -> (number=w752:dbl)  [unwired: 3 out]
                        n253 = property class="Slide (strict)"(reference=w754, error in=w756, "Value"=w752) -> (error out=w755:errorcluster)  [unwired: 1 out]
                      }
                      frame "Minimum" {
                        n254 = Fract/Exp String To Number(string=w759, default (0 dbl)=0.0 ("Data Range:Minimum")) -> (number=w757:dbl)  [unwired: 3 out]
                        n255 = property class="Slide (strict)"(reference=w760, error in=w762, "Data Range:Minimum"=w757) -> (error out=w761:errorcluster)  [unwired: 1 out]
                      }
                      frame "Scale.Minimum" {
                        n256 = Fract/Exp String To Number(string=w765, default (0 dbl)=0.0 ("Data Range:Minimum")) -> (number=w763:dbl)  [unwired: 3 out]
                        n257 = property class="Slide (strict)"(reference=w766, error in=w768, "Scale.Range:Minimum"=w763) -> (error out=w767:errorcluster)  [unwired: 1 out]
                      }
                      frame "Maximum" {
                        n258 = Fract/Exp String To Number(string=w771, default (0 dbl)=0.0 ("Data Range:Minimum")) -> (number=w769:dbl)  [unwired: 3 out]
                        n259 = property class="Slide (strict)"(reference=w772, error in=w774, "Data Range:Maximum"=w769) -> (error out=w773:errorcluster)  [unwired: 1 out]
                      }
                      frame "Scale.Maximum" {
                        n260 = Fract/Exp String To Number(string=w777, default (0 dbl)=0.0 ("Data Range:Minimum")) -> (number=w775:dbl)  [unwired: 3 out]
                        n261 = property class="Slide (strict)"(reference=w778, error in=w780, "Scale.Range:Maximum"=w775) -> (error out=w779:errorcluster)  [unwired: 1 out]
                      }
                      frame "Increment" {
                        n262 = Fract/Exp String To Number(string=w783, default (0 dbl)=0.0 ("Data Range:Minimum")) -> (number=w781:dbl)  [unwired: 3 out]
                        n263 = property class="Slide (strict)"(reference=w784, error in=w786, "Data Range:Increment"=w781) -> (error out=w785:errorcluster)  [unwired: 1 out]
                      }
                      frame "Scale.Increment" {
                        n264 = Fract/Exp String To Number(string=w789, default (0 dbl)=0.0 ("Data Range:Minimum")) -> (number=w787:dbl)  [unwired: 3 out]
                        n265 = property class="Slide (strict)"(reference=w790, error in=w792, "Scale.Range:Increment"=w787) -> (error out=w791:errorcluster)  [unwired: 1 out]
                      }
                      frame "Scale.Start" {
                        n266 = Fract/Exp String To Number(string=w795, default (0 dbl)=0.0 ("Data Range:Minimum")) -> (number=w793:dbl)  [unwired: 3 out]
                        n267 = property class="Slide (strict)"(reference=w796, error in=w798, "Scale.Range:Start"=w793) -> (error out=w797:errorcluster)  [unwired: 1 out]
                      }
                      frame "Scale.MinorInc" {
                        n268 = Fract/Exp String To Number(string=w801, default (0 dbl)=0.0 ("Data Range:Minimum")) -> (number=w799:dbl)  [unwired: 3 out]
                        n269 = property class="Slide (strict)"(reference=w802, error in=w804, "Scale.Range:Minor Increment"=w799) -> (error out=w803:errorcluster)  [unwired: 1 out]
                      }
                      frame "Scale.Format String" {
                        n270 = property class="Slide (strict)"(reference=w806, error in=w808, "Scale.Format String"=w805) -> (error out=w807:errorcluster)  [unwired: 1 out]
                      }
                      frame "Scale.Format" {
                        n271 = Decimal String To Number(string=w811, default (0L)=u8 0 ("Format & Precision:Format")) -> (number=w809:u8)  [unwired: 2 out]
                        n272 = property class="Slide (strict)"(reference=w812, error in=w814, "Scale.Format & Precision:Format"=w809) -> (error out=w813:errorcluster)  [unwired: 1 out]
                      }
                      frame "Scale.Precision" {
                        n273 = Decimal String To Number(string=w817, default (0L)=u8 0 ("Format & Precision:Format")) -> (number=w815:u8)  [unwired: 2 out]
                        n274 = property class="Slide (strict)"(reference=w818, error in=w820, "Scale.Format & Precision:Precision"=w815) -> (error out=w819:errorcluster)  [unwired: 1 out]
                      }
                    }
                  }
                  frame 11 {
                    n275 = Type Cast(type=refnum<vi> refnum ("Slide"), x=w827) -> (*(type *) &x=w824:refnum<vi>)
                    n276 = case shown="\"Value\"" w825 {
                      tunnel: w823 -> [w828 w834 w840 w846 w852 w858 w864 w870 w876 w882 w886 w892 w898]
                      tunnel: [w828 w833 w839 w845 w851 w857 w863 w869 w875 w881 w885 w891 w897] -> w821
                      tunnel: w824 -> [_ w832 w838 w844 w850 w856 w862 w868 w874 w880 w884 w890 w896]
                      tunnel: w822 -> [_ w831 w837 w843 w849 w855 w861 w867 w873 w879 w883 w889 w895]
                      frame "False", Default {
                      }
                      frame "Value" {
                        n277 = Fract/Exp String To Number(string=w831, default (0 dbl)=ext 0.0) -> (number=w830:ext)  [unwired: 3 out]
                        n278 = property class="Slide (strict)"(reference=w832, error in=w834, "Value"=w830) -> (error out=w833:errorcluster)  [unwired: 1 out]
                      }
                      frame "Minimum" {
                        n279 = Fract/Exp String To Number(string=w837, default (0 dbl)=0.0 ("Data Range:Minimum")) -> (number=w835:dbl)  [unwired: 3 out]
                        n280 = property class="Slide (strict)"(reference=w838, error in=w840, "Data Range:Minimum"=w835) -> (error out=w839:errorcluster)  [unwired: 1 out]
                      }
                      frame "Scale.Minimum" {
                        n281 = Fract/Exp String To Number(string=w843, default (0 dbl)=0.0 ("Data Range:Minimum")) -> (number=w841:dbl)  [unwired: 3 out]
                        n282 = property class="Slide (strict)"(reference=w844, error in=w846, "Scale.Range:Minimum"=w841) -> (error out=w845:errorcluster)  [unwired: 1 out]
                      }
                      frame "Maximum" {
                        n283 = Fract/Exp String To Number(string=w849, default (0 dbl)=0.0 ("Data Range:Minimum")) -> (number=w847:dbl)  [unwired: 3 out]
                        n284 = property class="Slide (strict)"(reference=w850, error in=w852, "Data Range:Maximum"=w847) -> (error out=w851:errorcluster)  [unwired: 1 out]
                      }
                      frame "Scale.Maximum" {
                        n285 = Fract/Exp String To Number(string=w855, default (0 dbl)=0.0 ("Data Range:Minimum")) -> (number=w853:dbl)  [unwired: 3 out]
                        n286 = property class="Slide (strict)"(reference=w856, error in=w858, "Scale.Range:Maximum"=w853) -> (error out=w857:errorcluster)  [unwired: 1 out]
                      }
                      frame "Increment" {
                        n287 = Fract/Exp String To Number(string=w861, default (0 dbl)=0.0 ("Data Range:Minimum")) -> (number=w859:dbl)  [unwired: 3 out]
                        n288 = property class="Slide (strict)"(reference=w862, error in=w864, "Data Range:Increment"=w859) -> (error out=w863:errorcluster)  [unwired: 1 out]
                      }
                      frame "Scale.Increment" {
                        n289 = Fract/Exp String To Number(string=w867, default (0 dbl)=0.0 ("Data Range:Minimum")) -> (number=w865:dbl)  [unwired: 3 out]
                        n290 = property class="Slide (strict)"(reference=w868, error in=w870, "Scale.Range:Increment"=w865) -> (error out=w869:errorcluster)  [unwired: 1 out]
                      }
                      frame "Scale.Start" {
                        n291 = Fract/Exp String To Number(string=w873, default (0 dbl)=0.0 ("Data Range:Minimum")) -> (number=w871:dbl)  [unwired: 3 out]
                        n292 = property class="Slide (strict)"(reference=w874, error in=w876, "Scale.Range:Start"=w871) -> (error out=w875:errorcluster)  [unwired: 1 out]
                      }
                      frame "Scale.MinorInc" {
                        n293 = Fract/Exp String To Number(string=w879, default (0 dbl)=0.0 ("Data Range:Minimum")) -> (number=w877:dbl)  [unwired: 3 out]
                        n294 = property class="Slide (strict)"(reference=w880, error in=w882, "Scale.Range:Minor Increment"=w877) -> (error out=w881:errorcluster)  [unwired: 1 out]
                      }
                      frame "Scale.Format String" {
                        n295 = property class="Slide (strict)"(reference=w884, error in=w886, "Scale.Format String"=w883) -> (error out=w885:errorcluster)  [unwired: 1 out]
                      }
                      frame "Scale.Format" {
                        n296 = Decimal String To Number(string=w889, default (0L)=u8 0 ("Format & Precision:Format")) -> (number=w887:u8)  [unwired: 2 out]
                        n297 = property class="Slide (strict)"(reference=w890, error in=w892, "Scale.Format & Precision:Format"=w887) -> (error out=w891:errorcluster)  [unwired: 1 out]
                      }
                      frame "Scale.Precision" {
                        n298 = Decimal String To Number(string=w895, default (0L)=u8 0 ("Format & Precision:Format")) -> (number=w893:u8)  [unwired: 2 out]
                        n299 = property class="Slide (strict)"(reference=w896, error in=w898, "Scale.Format & Precision:Precision"=w893) -> (error out=w897:errorcluster)  [unwired: 1 out]
                      }
                    }
                  }
                  frame 1 {
                    n300 = Type Cast(type=refnum<vi> refnum ("Slide"), x=w905) -> (*(type *) &x=w903:refnum<vi>)
                    n301 = case shown="\"Value\"" w904 {
                      tunnel: w901 -> [w906 w912 w918 w924 w930 w936 w942 w948 w954 w960 w964 w970 w976]
                      tunnel: [w906 w911 w917 w923 w929 w935 w941 w947 w953 w959 w963 w969 w975] -> w902
                      tunnel: w903 -> [_ w910 w916 w922 w928 w934 w940 w946 w952 w958 w962 w968 w974]
                      tunnel: w900 -> [_ w909 w915 w921 w927 w933 w939 w945 w951 w957 w961 w967 w973]
                      frame "False", Default {
                      }
                      frame "Value" {
                        n302 = Fract/Exp String To Number(string=w909, default (0 dbl)=u8 0) -> (number=w908:u8)  [unwired: 3 out]
                        n303 = property class="Slide (strict)"(reference=w910, error in=w912, "Value"=w908) -> (error out=w911:errorcluster)  [unwired: 1 out]
                      }
                      frame "Minimum" {
                        n304 = Fract/Exp String To Number(string=w915, default (0 dbl)=0.0 ("Data Range:Minimum")) -> (number=w913:dbl)  [unwired: 3 out]
                        n305 = property class="Slide (strict)"(reference=w916, error in=w918, "Data Range:Minimum"=w913) -> (error out=w917:errorcluster)  [unwired: 1 out]
                      }
                      frame "Scale.Minimum" {
                        n306 = Fract/Exp String To Number(string=w921, default (0 dbl)=0.0 ("Data Range:Minimum")) -> (number=w919:dbl)  [unwired: 3 out]
                        n307 = property class="Slide (strict)"(reference=w922, error in=w924, "Scale.Range:Minimum"=w919) -> (error out=w923:errorcluster)  [unwired: 1 out]
                      }
                      frame "Maximum" {
                        n308 = Fract/Exp String To Number(string=w927, default (0 dbl)=0.0 ("Data Range:Minimum")) -> (number=w925:dbl)  [unwired: 3 out]
                        n309 = property class="Slide (strict)"(reference=w928, error in=w930, "Data Range:Maximum"=w925) -> (error out=w929:errorcluster)  [unwired: 1 out]
                      }
                      frame "Scale.Maximum" {
                        n310 = Fract/Exp String To Number(string=w933, default (0 dbl)=0.0 ("Data Range:Minimum")) -> (number=w931:dbl)  [unwired: 3 out]
                        n311 = property class="Slide (strict)"(reference=w934, error in=w936, "Scale.Range:Maximum"=w931) -> (error out=w935:errorcluster)  [unwired: 1 out]
                      }
                      frame "Increment" {
                        n312 = Fract/Exp String To Number(string=w939, default (0 dbl)=0.0 ("Data Range:Minimum")) -> (number=w937:dbl)  [unwired: 3 out]
                        n313 = property class="Slide (strict)"(reference=w940, error in=w942, "Data Range:Increment"=w937) -> (error out=w941:errorcluster)  [unwired: 1 out]
                      }
                      frame "Scale.Increment" {
                        n314 = Fract/Exp String To Number(string=w945, default (0 dbl)=0.0 ("Data Range:Minimum")) -> (number=w943:dbl)  [unwired: 3 out]
                        n315 = property class="Slide (strict)"(reference=w946, error in=w948, "Scale.Range:Increment"=w943) -> (error out=w947:errorcluster)  [unwired: 1 out]
                      }
                      frame "Scale.Start" {
                        n316 = Fract/Exp String To Number(string=w951, default (0 dbl)=0.0 ("Data Range:Minimum")) -> (number=w949:dbl)  [unwired: 3 out]
                        n317 = property class="Slide (strict)"(reference=w952, error in=w954, "Scale.Range:Start"=w949) -> (error out=w953:errorcluster)  [unwired: 1 out]
                      }
                      frame "Scale.MinorInc" {
                        n318 = Fract/Exp String To Number(string=w957, default (0 dbl)=0.0 ("Data Range:Minimum")) -> (number=w955:dbl)  [unwired: 3 out]
                        n319 = property class="Slide (strict)"(reference=w958, error in=w960, "Scale.Range:Minor Increment"=w955) -> (error out=w959:errorcluster)  [unwired: 1 out]
                      }
                      frame "Scale.Format String" {
                        n320 = property class="Slide (strict)"(reference=w962, error in=w964, "Scale.Format String"=w961) -> (error out=w963:errorcluster)  [unwired: 1 out]
                      }
                      frame "Scale.Format" {
                        n321 = Decimal String To Number(string=w967, default (0L)=u8 0 ("Format & Precision:Format")) -> (number=w965:u8)  [unwired: 2 out]
                        n322 = property class="Slide (strict)"(reference=w968, error in=w970, "Scale.Format & Precision:Format"=w965) -> (error out=w969:errorcluster)  [unwired: 1 out]
                      }
                      frame "Scale.Precision" {
                        n323 = Decimal String To Number(string=w973, default (0L)=u8 0 ("Format & Precision:Format")) -> (number=w971:u8)  [unwired: 2 out]
                        n324 = property class="Slide (strict)"(reference=w974, error in=w976, "Scale.Format & Precision:Precision"=w971) -> (error out=w975:errorcluster)  [unwired: 1 out]
                      }
                    }
                  }
                  frame 2 {
                    n325 = Type Cast(type=refnum<vi> refnum ("Slide"), x=w983) -> (*(type *) &x=w980:refnum<vi>)
                    n326 = case shown="\"Value\"" w979 {
                      tunnel: w981 -> [w984 w990 w996 w1002 w1008 w1014 w1020 w1026 w1032 w1038 w1042 w1048 w1054]
                      tunnel: [w984 w989 w995 w1001 w1007 w1013 w1019 w1025 w1031 w1037 w1041 w1047 w1053] -> w982
                      tunnel: w980 -> [_ w988 w994 w1000 w1006 w1012 w1018 w1024 w1030 w1036 w1040 w1046 w1052]
                      tunnel: w978 -> [_ w987 w993 w999 w1005 w1011 w1017 w1023 w1029 w1035 w1039 w1045 w1051]
                      frame "False", Default {
                      }
                      frame "Value" {
                        n327 = Fract/Exp String To Number(string=w987, default (0 dbl)=u16 0) -> (number=w986:u16)  [unwired: 3 out]
                        n328 = property class="Slide (strict)"(reference=w988, error in=w990, "Value"=w986) -> (error out=w989:errorcluster)  [unwired: 1 out]
                      }
                      frame "Minimum" {
                        n329 = Fract/Exp String To Number(string=w993, default (0 dbl)=0.0 ("Data Range:Minimum")) -> (number=w991:dbl)  [unwired: 3 out]
                        n330 = property class="Slide (strict)"(reference=w994, error in=w996, "Data Range:Minimum"=w991) -> (error out=w995:errorcluster)  [unwired: 1 out]
                      }
                      frame "Scale.Minimum" {
                        n331 = Fract/Exp String To Number(string=w999, default (0 dbl)=0.0 ("Data Range:Minimum")) -> (number=w997:dbl)  [unwired: 3 out]
                        n332 = property class="Slide (strict)"(reference=w1000, error in=w1002, "Scale.Range:Minimum"=w997) -> (error out=w1001:errorcluster)  [unwired: 1 out]
                      }
                      frame "Maximum" {
                        n333 = Fract/Exp String To Number(string=w1005, default (0 dbl)=0.0 ("Data Range:Minimum")) -> (number=w1003:dbl)  [unwired: 3 out]
                        n334 = property class="Slide (strict)"(reference=w1006, error in=w1008, "Data Range:Maximum"=w1003) -> (error out=w1007:errorcluster)  [unwired: 1 out]
                      }
                      frame "Scale.Maximum" {
                        n335 = Fract/Exp String To Number(string=w1011, default (0 dbl)=0.0 ("Data Range:Minimum")) -> (number=w1009:dbl)  [unwired: 3 out]
                        n336 = property class="Slide (strict)"(reference=w1012, error in=w1014, "Scale.Range:Maximum"=w1009) -> (error out=w1013:errorcluster)  [unwired: 1 out]
                      }
                      frame "Increment" {
                        n337 = Fract/Exp String To Number(string=w1017, default (0 dbl)=0.0 ("Data Range:Minimum")) -> (number=w1015:dbl)  [unwired: 3 out]
                        n338 = property class="Slide (strict)"(reference=w1018, error in=w1020, "Data Range:Increment"=w1015) -> (error out=w1019:errorcluster)  [unwired: 1 out]
                      }
                      frame "Scale.Increment" {
                        n339 = Fract/Exp String To Number(string=w1023, default (0 dbl)=0.0 ("Data Range:Minimum")) -> (number=w1021:dbl)  [unwired: 3 out]
                        n340 = property class="Slide (strict)"(reference=w1024, error in=w1026, "Scale.Range:Increment"=w1021) -> (error out=w1025:errorcluster)  [unwired: 1 out]
                      }
                      frame "Scale.Start" {
                        n341 = Fract/Exp String To Number(string=w1029, default (0 dbl)=0.0 ("Data Range:Minimum")) -> (number=w1027:dbl)  [unwired: 3 out]
                        n342 = property class="Slide (strict)"(reference=w1030, error in=w1032, "Scale.Range:Start"=w1027) -> (error out=w1031:errorcluster)  [unwired: 1 out]
                      }
                      frame "Scale.MinorInc" {
                        n343 = Fract/Exp String To Number(string=w1035, default (0 dbl)=0.0 ("Data Range:Minimum")) -> (number=w1033:dbl)  [unwired: 3 out]
                        n344 = property class="Slide (strict)"(reference=w1036, error in=w1038, "Scale.Range:Minor Increment"=w1033) -> (error out=w1037:errorcluster)  [unwired: 1 out]
                      }
                      frame "Scale.Format String" {
                        n345 = property class="Slide (strict)"(reference=w1040, error in=w1042, "Scale.Format String"=w1039) -> (error out=w1041:errorcluster)  [unwired: 1 out]
                      }
                      frame "Scale.Format" {
                        n346 = Decimal String To Number(string=w1045, default (0L)=u8 0 ("Format & Precision:Format")) -> (number=w1043:u8)  [unwired: 2 out]
                        n347 = property class="Slide (strict)"(reference=w1046, error in=w1048, "Scale.Format & Precision:Format"=w1043) -> (error out=w1047:errorcluster)  [unwired: 1 out]
                      }
                      frame "Scale.Precision" {
                        n348 = Decimal String To Number(string=w1051, default (0L)=u8 0 ("Format & Precision:Format")) -> (number=w1049:u8)  [unwired: 2 out]
                        n349 = property class="Slide (strict)"(reference=w1052, error in=w1054, "Scale.Format & Precision:Precision"=w1049) -> (error out=w1053:errorcluster)  [unwired: 1 out]
                      }
                    }
                  }
                  frame 3 {
                    n350 = Type Cast(type=refnum<vi> refnum ("Slide"), x=w1061) -> (*(type *) &x=w1057:refnum<vi>)
                    n351 = case shown="\"Value\"" w1058 {
                      tunnel: [w1062 w1068 w1074 w1080 w1086 w1092 w1098 w1104 w1110 w1116 w1120 w1126 w1132] -> w1059
                      tunnel: w1057 -> [_ w1063 w1069 w1077 w1082 w1088 w1094 w1100 w1105 w1113 w1118 w1121 w1129]
                      tunnel: w1056 -> [w1062 w1065 w1071 w1076 w1081 w1089 w1095 w1101 w1107 w1112 w1119 w1123 w1127]
                      tunnel: w1055 -> [_ w1064 w1070 w1075 w1083 w1087 w1093 w1099 w1106 w1111 w1117 w1122 w1128]
                      frame "False", Default {
                      }
                      frame "Value" {
                        n352 = Fract/Exp String To Number(string=w1064, default (0 dbl)=0) -> (number=w1067:i32)  [unwired: 3 out]
                        n353 = property class="Slide (strict)"(reference=w1063, error in=w1065, "Value"=w1067) -> (error out=w1068:errorcluster)  [unwired: 1 out]
                      }
                      frame "Minimum" {
                        n354 = Fract/Exp String To Number(string=w1070, default (0 dbl)=0.0 ("Data Range:Minimum")) -> (number=w1072:dbl)  [unwired: 3 out]
                        n355 = property class="Slide (strict)"(reference=w1069, error in=w1071, "Data Range:Minimum"=w1072) -> (error out=w1074:errorcluster)  [unwired: 1 out]
                      }
                      frame "Scale.Minimum" {
                        n356 = Fract/Exp String To Number(string=w1075, default (0 dbl)=0.0 ("Data Range:Minimum")) -> (number=w1078:dbl)  [unwired: 3 out]
                        n357 = property class="Slide (strict)"(reference=w1077, error in=w1076, "Scale.Range:Minimum"=w1078) -> (error out=w1080:errorcluster)  [unwired: 1 out]
                      }
                      frame "Maximum" {
                        n358 = Fract/Exp String To Number(string=w1083, default (0 dbl)=0.0 ("Data Range:Minimum")) -> (number=w1084:dbl)  [unwired: 3 out]
                        n359 = property class="Slide (strict)"(reference=w1082, error in=w1081, "Data Range:Maximum"=w1084) -> (error out=w1086:errorcluster)  [unwired: 1 out]
                      }
                      frame "Scale.Maximum" {
                        n360 = Fract/Exp String To Number(string=w1087, default (0 dbl)=0.0 ("Data Range:Minimum")) -> (number=w1090:dbl)  [unwired: 3 out]
                        n361 = property class="Slide (strict)"(reference=w1088, error in=w1089, "Scale.Range:Maximum"=w1090) -> (error out=w1092:errorcluster)  [unwired: 1 out]
                      }
                      frame "Increment" {
                        n362 = Fract/Exp String To Number(string=w1093, default (0 dbl)=0.0 ("Data Range:Minimum")) -> (number=w1096:dbl)  [unwired: 3 out]
                        n363 = property class="Slide (strict)"(reference=w1094, error in=w1095, "Data Range:Increment"=w1096) -> (error out=w1098:errorcluster)  [unwired: 1 out]
                      }
                      frame "Scale.Increment" {
                        n364 = Fract/Exp String To Number(string=w1099, default (0 dbl)=0.0 ("Data Range:Minimum")) -> (number=w1102:dbl)  [unwired: 3 out]
                        n365 = property class="Slide (strict)"(reference=w1100, error in=w1101, "Scale.Range:Increment"=w1102) -> (error out=w1104:errorcluster)  [unwired: 1 out]
                      }
                      frame "Scale.Start" {
                        n366 = Fract/Exp String To Number(string=w1106, default (0 dbl)=0.0 ("Data Range:Minimum")) -> (number=w1108:dbl)  [unwired: 3 out]
                        n367 = property class="Slide (strict)"(reference=w1105, error in=w1107, "Scale.Range:Start"=w1108) -> (error out=w1110:errorcluster)  [unwired: 1 out]
                      }
                      frame "Scale.MinorInc" {
                        n368 = Fract/Exp String To Number(string=w1111, default (0 dbl)=0.0 ("Data Range:Minimum")) -> (number=w1114:dbl)  [unwired: 3 out]
                        n369 = property class="Slide (strict)"(reference=w1113, error in=w1112, "Scale.Range:Minor Increment"=w1114) -> (error out=w1116:errorcluster)  [unwired: 1 out]
                      }
                      frame "Scale.Format String" {
                        n370 = property class="Slide (strict)"(reference=w1118, error in=w1119, "Scale.Format String"=w1117) -> (error out=w1120:errorcluster)  [unwired: 1 out]
                      }
                      frame "Scale.Format" {
                        n371 = Decimal String To Number(string=w1122, default (0L)=u8 0 ("Format & Precision:Format")) -> (number=w1124:u8)  [unwired: 2 out]
                        n372 = property class="Slide (strict)"(reference=w1121, error in=w1123, "Scale.Format & Precision:Format"=w1124) -> (error out=w1126:errorcluster)  [unwired: 1 out]
                      }
                      frame "Scale.Precision" {
                        n373 = Decimal String To Number(string=w1128, default (0L)=u8 0 ("Format & Precision:Format")) -> (number=w1130:u8)  [unwired: 2 out]
                        n374 = property class="Slide (strict)"(reference=w1129, error in=w1127, "Scale.Format & Precision:Precision"=w1130) -> (error out=w1132:errorcluster)  [unwired: 1 out]
                      }
                    }
                  }
                  frame 5 {
                    n375 = Type Cast(type=refnum<vi> refnum ("Slide"), x=w1139) -> (*(type *) &x=w1136:refnum<vi>)
                    n376 = case shown="\"Value\"" w1137 {
                      tunnel: [w1140 w1146 w1152 w1158 w1164 w1170 w1176 w1182 w1188 w1194 w1198 w1204 w1210] -> w1133
                      tunnel: w1136 -> [_ w1141 w1147 w1155 w1160 w1166 w1172 w1178 w1183 w1191 w1196 w1199 w1207]
                      tunnel: w1135 -> [w1140 w1143 w1149 w1154 w1159 w1167 w1173 w1179 w1185 w1190 w1197 w1201 w1205]
                      tunnel: w1134 -> [_ w1142 w1148 w1153 w1161 w1165 w1171 w1177 w1184 w1189 w1195 w1200 w1206]
                      frame "False", Default {
                      }
                      frame "Value" {
                        n377 = Fract/Exp String To Number(string=w1142, default (0 dbl)=u8 0) -> (number=w1145:u8)  [unwired: 3 out]
                        n378 = property class="Slide (strict)"(reference=w1141, error in=w1143, "Value"=w1145) -> (error out=w1146:errorcluster)  [unwired: 1 out]
                      }
                      frame "Minimum" {
                        n379 = Fract/Exp String To Number(string=w1148, default (0 dbl)=0.0 ("Data Range:Minimum")) -> (number=w1150:dbl)  [unwired: 3 out]
                        n380 = property class="Slide (strict)"(reference=w1147, error in=w1149, "Data Range:Minimum"=w1150) -> (error out=w1152:errorcluster)  [unwired: 1 out]
                      }
                      frame "Scale.Minimum" {
                        n381 = Fract/Exp String To Number(string=w1153, default (0 dbl)=0.0 ("Data Range:Minimum")) -> (number=w1156:dbl)  [unwired: 3 out]
                        n382 = property class="Slide (strict)"(reference=w1155, error in=w1154, "Scale.Range:Minimum"=w1156) -> (error out=w1158:errorcluster)  [unwired: 1 out]
                      }
                      frame "Maximum" {
                        n383 = Fract/Exp String To Number(string=w1161, default (0 dbl)=0.0 ("Data Range:Minimum")) -> (number=w1162:dbl)  [unwired: 3 out]
                        n384 = property class="Slide (strict)"(reference=w1160, error in=w1159, "Data Range:Maximum"=w1162) -> (error out=w1164:errorcluster)  [unwired: 1 out]
                      }
                      frame "Scale.Maximum" {
                        n385 = Fract/Exp String To Number(string=w1165, default (0 dbl)=0.0 ("Data Range:Minimum")) -> (number=w1168:dbl)  [unwired: 3 out]
                        n386 = property class="Slide (strict)"(reference=w1166, error in=w1167, "Scale.Range:Maximum"=w1168) -> (error out=w1170:errorcluster)  [unwired: 1 out]
                      }
                      frame "Increment" {
                        n387 = Fract/Exp String To Number(string=w1171, default (0 dbl)=0.0 ("Data Range:Minimum")) -> (number=w1174:dbl)  [unwired: 3 out]
                        n388 = property class="Slide (strict)"(reference=w1172, error in=w1173, "Data Range:Increment"=w1174) -> (error out=w1176:errorcluster)  [unwired: 1 out]
                      }
                      frame "Scale.Increment" {
                        n389 = Fract/Exp String To Number(string=w1177, default (0 dbl)=0.0 ("Data Range:Minimum")) -> (number=w1180:dbl)  [unwired: 3 out]
                        n390 = property class="Slide (strict)"(reference=w1178, error in=w1179, "Scale.Range:Increment"=w1180) -> (error out=w1182:errorcluster)  [unwired: 1 out]
                      }
                      frame "Scale.Start" {
                        n391 = Fract/Exp String To Number(string=w1184, default (0 dbl)=0.0 ("Data Range:Minimum")) -> (number=w1186:dbl)  [unwired: 3 out]
                        n392 = property class="Slide (strict)"(reference=w1183, error in=w1185, "Scale.Range:Start"=w1186) -> (error out=w1188:errorcluster)  [unwired: 1 out]
                      }
                      frame "Scale.MinorInc" {
                        n393 = Fract/Exp String To Number(string=w1189, default (0 dbl)=0.0 ("Data Range:Minimum")) -> (number=w1192:dbl)  [unwired: 3 out]
                        n394 = property class="Slide (strict)"(reference=w1191, error in=w1190, "Scale.Range:Minor Increment"=w1192) -> (error out=w1194:errorcluster)  [unwired: 1 out]
                      }
                      frame "Scale.Format String" {
                        n395 = property class="Slide (strict)"(reference=w1196, error in=w1197, "Scale.Format String"=w1195) -> (error out=w1198:errorcluster)  [unwired: 1 out]
                      }
                      frame "Scale.Format" {
                        n396 = Decimal String To Number(string=w1200, default (0L)=u8 0 ("Format & Precision:Format")) -> (number=w1202:u8)  [unwired: 2 out]
                        n397 = property class="Slide (strict)"(reference=w1199, error in=w1201, "Scale.Format & Precision:Format"=w1202) -> (error out=w1204:errorcluster)  [unwired: 1 out]
                      }
                      frame "Scale.Precision" {
                        n398 = Decimal String To Number(string=w1206, default (0L)=u8 0 ("Format & Precision:Format")) -> (number=w1208:u8)  [unwired: 2 out]
                        n399 = property class="Slide (strict)"(reference=w1207, error in=w1205, "Scale.Format & Precision:Precision"=w1208) -> (error out=w1210:errorcluster)  [unwired: 1 out]
                      }
                    }
                  }
                  frame 6 {
                    n400 = Type Cast(type=refnum<vi> refnum ("Slide"), x=w1217) -> (*(type *) &x=w1214:refnum<vi>)
                    n401 = case shown="\"Value\"" w1215 {
                      tunnel: [w1218 w1224 w1230 w1236 w1242 w1248 w1254 w1260 w1266 w1272 w1276 w1282 w1288] -> w1213
                      tunnel: w1214 -> [_ w1219 w1225 w1233 w1238 w1244 w1250 w1256 w1261 w1269 w1274 w1277 w1285]
                      tunnel: w1212 -> [w1218 w1221 w1227 w1232 w1237 w1245 w1251 w1257 w1263 w1268 w1275 w1279 w1283]
                      tunnel: w1211 -> [_ w1220 w1226 w1231 w1239 w1243 w1249 w1255 w1262 w1267 w1273 w1278 w1284]
                      frame "False", Default {
                      }
                      frame "Value" {
                        n402 = Fract/Exp String To Number(string=w1220, default (0 dbl)=u16 0) -> (number=w1223:u16)  [unwired: 3 out]
                        n403 = property class="Slide (strict)"(reference=w1219, error in=w1221, "Value"=w1223) -> (error out=w1224:errorcluster)  [unwired: 1 out]
                      }
                      frame "Minimum" {
                        n404 = Fract/Exp String To Number(string=w1226, default (0 dbl)=0.0 ("Data Range:Minimum")) -> (number=w1228:dbl)  [unwired: 3 out]
                        n405 = property class="Slide (strict)"(reference=w1225, error in=w1227, "Data Range:Minimum"=w1228) -> (error out=w1230:errorcluster)  [unwired: 1 out]
                      }
                      frame "Scale.Minimum" {
                        n406 = Fract/Exp String To Number(string=w1231, default (0 dbl)=0.0 ("Data Range:Minimum")) -> (number=w1234:dbl)  [unwired: 3 out]
                        n407 = property class="Slide (strict)"(reference=w1233, error in=w1232, "Scale.Range:Minimum"=w1234) -> (error out=w1236:errorcluster)  [unwired: 1 out]
                      }
                      frame "Maximum" {
                        n408 = Fract/Exp String To Number(string=w1239, default (0 dbl)=0.0 ("Data Range:Minimum")) -> (number=w1240:dbl)  [unwired: 3 out]
                        n409 = property class="Slide (strict)"(reference=w1238, error in=w1237, "Data Range:Maximum"=w1240) -> (error out=w1242:errorcluster)  [unwired: 1 out]
                      }
                      frame "Scale.Maximum" {
                        n410 = Fract/Exp String To Number(string=w1243, default (0 dbl)=0.0 ("Data Range:Minimum")) -> (number=w1246:dbl)  [unwired: 3 out]
                        n411 = property class="Slide (strict)"(reference=w1244, error in=w1245, "Scale.Range:Maximum"=w1246) -> (error out=w1248:errorcluster)  [unwired: 1 out]
                      }
                      frame "Increment" {
                        n412 = Fract/Exp String To Number(string=w1249, default (0 dbl)=0.0 ("Data Range:Minimum")) -> (number=w1252:dbl)  [unwired: 3 out]
                        n413 = property class="Slide (strict)"(reference=w1250, error in=w1251, "Data Range:Increment"=w1252) -> (error out=w1254:errorcluster)  [unwired: 1 out]
                      }
                      frame "Scale.Increment" {
                        n414 = Fract/Exp String To Number(string=w1255, default (0 dbl)=0.0 ("Data Range:Minimum")) -> (number=w1258:dbl)  [unwired: 3 out]
                        n415 = property class="Slide (strict)"(reference=w1256, error in=w1257, "Scale.Range:Increment"=w1258) -> (error out=w1260:errorcluster)  [unwired: 1 out]
                      }
                      frame "Scale.Start" {
                        n416 = Fract/Exp String To Number(string=w1262, default (0 dbl)=0.0 ("Data Range:Minimum")) -> (number=w1264:dbl)  [unwired: 3 out]
                        n417 = property class="Slide (strict)"(reference=w1261, error in=w1263, "Scale.Range:Start"=w1264) -> (error out=w1266:errorcluster)  [unwired: 1 out]
                      }
                      frame "Scale.MinorInc" {
                        n418 = Fract/Exp String To Number(string=w1267, default (0 dbl)=0.0 ("Data Range:Minimum")) -> (number=w1270:dbl)  [unwired: 3 out]
                        n419 = property class="Slide (strict)"(reference=w1269, error in=w1268, "Scale.Range:Minor Increment"=w1270) -> (error out=w1272:errorcluster)  [unwired: 1 out]
                      }
                      frame "Scale.Format String" {
                        n420 = property class="Slide (strict)"(reference=w1274, error in=w1275, "Scale.Format String"=w1273) -> (error out=w1276:errorcluster)  [unwired: 1 out]
                      }
                      frame "Scale.Format" {
                        n421 = Decimal String To Number(string=w1278, default (0L)=u8 0 ("Format & Precision:Format")) -> (number=w1280:u8)  [unwired: 2 out]
                        n422 = property class="Slide (strict)"(reference=w1277, error in=w1279, "Scale.Format & Precision:Format"=w1280) -> (error out=w1282:errorcluster)  [unwired: 1 out]
                      }
                      frame "Scale.Precision" {
                        n423 = Decimal String To Number(string=w1284, default (0L)=u8 0 ("Format & Precision:Format")) -> (number=w1286:u8)  [unwired: 2 out]
                        n424 = property class="Slide (strict)"(reference=w1285, error in=w1283, "Scale.Format & Precision:Precision"=w1286) -> (error out=w1288:errorcluster)  [unwired: 1 out]
                      }
                    }
                  }
                  frame 7 {
                    n425 = Type Cast(type=refnum<vi> refnum ("Slide"), x=w1295) -> (*(type *) &x=w1292:refnum<vi>)
                    n426 = case shown="\"Value\"" w1293 {
                      tunnel: [w1296 w1302 w1308 w1314 w1320 w1326 w1332 w1338 w1344 w1350 w1354 w1360 w1366] -> w1289
                      tunnel: w1292 -> [_ w1297 w1303 w1311 w1316 w1322 w1328 w1334 w1339 w1347 w1352 w1355 w1363]
                      tunnel: w1291 -> [w1296 w1299 w1305 w1310 w1315 w1323 w1329 w1335 w1341 w1346 w1353 w1357 w1361]
                      tunnel: w1290 -> [_ w1298 w1304 w1309 w1317 w1321 w1327 w1333 w1340 w1345 w1351 w1356 w1362]
                      frame "False", Default {
                      }
                      frame "Value" {
                        n427 = Fract/Exp String To Number(string=w1298, default (0 dbl)=u32 0) -> (number=w1301:u32)  [unwired: 3 out]
                        n428 = property class="Slide (strict)"(reference=w1297, error in=w1299, "Value"=w1301) -> (error out=w1302:errorcluster)  [unwired: 1 out]
                      }
                      frame "Minimum" {
                        n429 = Fract/Exp String To Number(string=w1304, default (0 dbl)=0.0 ("Data Range:Minimum")) -> (number=w1306:dbl)  [unwired: 3 out]
                        n430 = property class="Slide (strict)"(reference=w1303, error in=w1305, "Data Range:Minimum"=w1306) -> (error out=w1308:errorcluster)  [unwired: 1 out]
                      }
                      frame "Scale.Minimum" {
                        n431 = Fract/Exp String To Number(string=w1309, default (0 dbl)=0.0 ("Data Range:Minimum")) -> (number=w1312:dbl)  [unwired: 3 out]
                        n432 = property class="Slide (strict)"(reference=w1311, error in=w1310, "Scale.Range:Minimum"=w1312) -> (error out=w1314:errorcluster)  [unwired: 1 out]
                      }
                      frame "Maximum" {
                        n433 = Fract/Exp String To Number(string=w1317, default (0 dbl)=0.0 ("Data Range:Minimum")) -> (number=w1318:dbl)  [unwired: 3 out]
                        n434 = property class="Slide (strict)"(reference=w1316, error in=w1315, "Data Range:Maximum"=w1318) -> (error out=w1320:errorcluster)  [unwired: 1 out]
                      }
                      frame "Scale.Maximum" {
                        n435 = Fract/Exp String To Number(string=w1321, default (0 dbl)=0.0 ("Data Range:Minimum")) -> (number=w1324:dbl)  [unwired: 3 out]
                        n436 = property class="Slide (strict)"(reference=w1322, error in=w1323, "Scale.Range:Maximum"=w1324) -> (error out=w1326:errorcluster)  [unwired: 1 out]
                      }
                      frame "Increment" {
                        n437 = Fract/Exp String To Number(string=w1327, default (0 dbl)=0.0 ("Data Range:Minimum")) -> (number=w1330:dbl)  [unwired: 3 out]
                        n438 = property class="Slide (strict)"(reference=w1328, error in=w1329, "Data Range:Increment"=w1330) -> (error out=w1332:errorcluster)  [unwired: 1 out]
                      }
                      frame "Scale.Increment" {
                        n439 = Fract/Exp String To Number(string=w1333, default (0 dbl)=0.0 ("Data Range:Minimum")) -> (number=w1336:dbl)  [unwired: 3 out]
                        n440 = property class="Slide (strict)"(reference=w1334, error in=w1335, "Scale.Range:Increment"=w1336) -> (error out=w1338:errorcluster)  [unwired: 1 out]
                      }
                      frame "Scale.Start" {
                        n441 = Fract/Exp String To Number(string=w1340, default (0 dbl)=0.0 ("Data Range:Minimum")) -> (number=w1342:dbl)  [unwired: 3 out]
                        n442 = property class="Slide (strict)"(reference=w1339, error in=w1341, "Scale.Range:Start"=w1342) -> (error out=w1344:errorcluster)  [unwired: 1 out]
                      }
                      frame "Scale.MinorInc" {
                        n443 = Fract/Exp String To Number(string=w1345, default (0 dbl)=0.0 ("Data Range:Minimum")) -> (number=w1348:dbl)  [unwired: 3 out]
                        n444 = property class="Slide (strict)"(reference=w1347, error in=w1346, "Scale.Range:Minor Increment"=w1348) -> (error out=w1350:errorcluster)  [unwired: 1 out]
                      }
                      frame "Scale.Format String" {
                        n445 = property class="Slide (strict)"(reference=w1352, error in=w1353, "Scale.Format String"=w1351) -> (error out=w1354:errorcluster)  [unwired: 1 out]
                      }
                      frame "Scale.Format" {
                        n446 = Decimal String To Number(string=w1356, default (0L)=u8 0 ("Format & Precision:Format")) -> (number=w1358:u8)  [unwired: 2 out]
                        n447 = property class="Slide (strict)"(reference=w1355, error in=w1357, "Scale.Format & Precision:Format"=w1358) -> (error out=w1360:errorcluster)  [unwired: 1 out]
                      }
                      frame "Scale.Precision" {
                        n448 = Decimal String To Number(string=w1362, default (0L)=u8 0 ("Format & Precision:Format")) -> (number=w1364:u8)  [unwired: 2 out]
                        n449 = property class="Slide (strict)"(reference=w1363, error in=w1361, "Scale.Format & Precision:Precision"=w1364) -> (error out=w1366:errorcluster)  [unwired: 1 out]
                      }
                    }
                  }
                }
              }
              frame "Boolean" {
                n450 = Type Cast(type=refnum<vi> refnum ("Boolean 2"), x=w1371) -> (*(type *) &x=w1370:refnum<vi>)
                n451 = case shown="\"Value\"" w1367 {
                  tunnel: w1373 -> [w1374 w1380 w1384]
                  tunnel: [w1374 w1379 w1383] -> w1372
                  tunnel: w1370 -> [_ w1378 w1382]
                  tunnel: w1369 -> [_ w1376 w1381]
                  frame "False", Default {
                  }
                  frame "Value" {
                    n452 = Equal?(x=w1376, y="TRUE" ("x")) -> (x = y?=w1377:bool)
                    n453 = property class="Bool (strict)"(reference=w1378, error in=w1380, "Value"=w1377) -> (error out=w1379:errorcluster)  [unwired: 1 out]
                  }
                  frame "BooleanText" {
                    n454 = property class="Bool (strict)"(reference=w1382, error in=w1384, "Boolean Text.Text"=w1381) -> (error out=w1383:errorcluster)  [unwired: 1 out]
                  }
                }
              }
            }
          }
          frame -1 {
          }
        }
      }
      n455 = case shown="True" w24 {
        tunnel: [w1387 w1392] -> w26
        tunnel: w18 -> [w1387 w1391]
        tunnel: w13 -> [w1386 w1390]
        tunnel: [w1386 w1388] -> w25
        frame False {
        }
        frame True {
          n456 = call "VI Server_Defer FP Update.vi"("Defer Panel Updates? (F)"=FALSE ("Defer Panel Updates (F)"), "error in"=w1391, "VI Server Cluster"=w1390) -> ("error out"=w1392:errorcluster, "VI Server Cluster.DUP"=w1388:T1)  [unwired: 7 out]
        }
      }
      n457 = call "VI Server_Empty VI Server Cluster.vi"() -> ("VI Server Cluster"=w12:T1)  [unwired: 7 in]
    }
    frame Error {
    }
  }
  "error out" <- w9
  "Labels.Text" <- w5
  "VI Server Cluster.DUP" <- w4
  n458 = local write "VI Server Cluster"(w1) -> ()
  n459 = Request Deallocation(w2) -> ()
